vi "GUI.vi"() -> ()   [LabVIEW 2023]
uses:
  <vilib>/userDefined/High Color/IMAQdx.ctl
  <vilib>/vision/Image Controls.llb/IMAQ Image.ctl
  <vilib>/vision/Avi.llb/IMAQ AVI2 Refnum.ctl
  <vilib>/vision/driver/IMAQdx.llb/IMAQdx Acquisition Mode.ctl
  <vilib>/vision/driver/IMAQdx.llb/IMAQdx Buffer Number Mode.ctl
  <vilib>/Utility/error.llb/DialogType.ctl
  <vilib>/DAQmx/write.llb/DAQmx Write (Analog 1D Wfm NChan NSamp).vi
  <extravilib>/ChannelInstances/Tag-bool/Read With Abort.vi
  <extravilib>/ChannelInstances/Tag-t'IMAQ Image.ctl'/Read With Abort.vi
  <extravilib>/ChannelInstances/Messenger-str/Write With Abort.vi
  <extravilib>/ChannelInstances/Tag-str/Read With Abort.vi
  <extravilib>/ChannelInstances/Messenger-str/Read With Abort.vi
  <extravilib>/ChannelInstances/Tag-str/Write With Abort.vi
  <extravilib>/ChannelInstances/Tag-bool/Write With Abort.vi
  <extravilib>/ChannelInstances/Messenger-c(bool,i32,str)/Read With Abort.vi
  <extravilib>/ChannelInstances/Tag-c(bool,i32,str)/Write With Abort.vi
  <extravilib>/ChannelInstances/Tag-c(bool,i32,str)/Read With Abort.vi
  <extravilib>/ChannelInstances/Messenger-c(bool,i32,str)/Write With Abort.vi
  <vilib>/Utility/High Resolution Relative Seconds.vi
  <extravilib>/ChannelInstances/Tag-t'IMAQ Image.ctl'/Write With Abort.vi
  <extravilib>/ChannelInstances/Tag-str/Instantiate.vi
  <extravilib>/ChannelInstances/Messenger-str/Instantiate.vi
  <vilib>/DAQmx/create/channels.llb/DAQmx Create Channel (AO-Voltage-Basic).vi
  <vilib>/DAQmx/configure/timing.llb/DAQmx Timing (Sample Clock).vi
  <vilib>/DAQmx/configure/trigger.llb/DAQmx Start Trigger (Digital Edge).vi
  <vilib>/DAQmx/miscellaneous.llb/DAQmx Fill In Error Info.vi
  <extravilib>/ChannelInstances/Messenger-str/Endpoint.vi
  <extravilib>/ChannelInstances/Tag-str/EndpointRead.vi
  <extravilib>/ChannelInstances/Tag-str/Endpoint.vi
  <extravilib>/ChannelInstances/Tag-bool/Instantiate.vi
  <extravilib>/ChannelInstances/Tag-bool/Endpoint.vi
  <extravilib>/ChannelInstances/Tag-t'IMAQ Image.ctl'/Instantiate.vi
  <extravilib>/ChannelInstances/Tag-bool/EndpointRead.vi
  <extravilib>/ChannelInstances/Tag-t'IMAQ Image.ctl'/EndpointRead.vi
  <extravilib>/ChannelInstances/Tag-c(bool,i32,str)/Instantiate.vi
  <extravilib>/ChannelInstances/Messenger-c(bool,i32,str)/Instantiate.vi
  <extravilib>/ChannelInstances/Messenger-c(bool,i32,str)/Endpoint.vi
  <extravilib>/ChannelInstances/Tag-c(bool,i32,str)/Endpoint.vi
  <extravilib>/ChannelInstances/Tag-c(bool,i32,str)/EndpointRead.vi
  <vilib>/vision/EDVR.llb/IMAQ ImageToEDVR.vi
  <vilib>/vision/EDVR.llb/IMAQ ImageToEDVR 1D U8.vi
  <vilib>/vision/EDVR.llb/IMAQ ImageToEDVR 1D I16.vi
  <vilib>/vision/EDVR.llb/IMAQ ImageToEDVR 1D U32.vi
  <vilib>/vision/EDVR.llb/IMAQ ImageToEDVR 1D U16.vi
  <extravilib>/ChannelInstances/Tag-t'IMAQ Image.ctl'/Endpoint.vi
  <vilib>/vision/driver/NI_Vision_Acquisition_Software.lvlib
  <resource>/objmgr/imaqdx.rc
  <extravilib>/ChannelInstances/Messenger-str.lvlib
  <extravilib>/ChannelInstances/Messenger-c(bool,i32,str).lvlib
  <extravilib>/ChannelInstances/Tag-c(bool,i32,str).lvlib
  <extravilib>/ChannelInstances/Tag-t'IMAQ Image.ctl'.lvlib
  <extravilib>/ChannelInstances/Tag-bool.lvlib
  <resource>/objmgr/daqmx.rc
  <extravilib>/ChannelInstances/Tag-str.lvlib
  Control2.ctl
panel:
  in  "error IO":errorcluster
  in  "Stop 7":bool
  in  "Stop 6":bool
  in  "Stop 5":bool
  in  "Stop 4":bool
  in  "Stop 3":bool
  in  "Stop 2":bool
  in  "Stop":bool
  in  "Save Name":string
  in  "Save Path":path
  in  "Save Config":bool
  in  "Apply Configuration":bool
  in  "Config Path":path
  in  "Initialize from config file?":bool caption="Checkbox"
  in  "Quit":bool
  in  "Clock Button":bool
  in  "Controls":bool
  in  "Inputs":bool
  in  "Outputs":bool
  in  "Camera Setup":bool
  out "Tab Control":T1(tab)
  out "Sensor Readout Time":dbl
  out "Max FPS":dbl
  out "FPS":dbl
  out "Images Behind":dbl
  out "Missed Images":dbl
  out "Video Bytes/s":dbl
  out "Estimated Time":dbl
  in  "Initialize Camera":bool
  in  "Cluster - Borderless":T3={"Cluster - Borderless"={"Time Stamp\n Position"=enum."Exposure Center", "Frame rate Multiple of \nData Acquisition Rate"=FALSE}, "Sensor readout mode\n(Fast Decreases Quality)"=enum."Normal", "Pixel Format\n(p not supported)"=enum."Mono 10 p", "Gain"=0.0, "Gamma"=1.0, "Temporary Format\n(can be converted)"=enum."AVI", "Cluster - Borderless 2"={"Frame Limit"=0.0}, "Cluster - Borderless 3"={"Frame Limit"=0.0}, "Camera Ref"="", "Tempory Storage Location\n(File can be moved after acquisition)\nSSD recomended for high frame rate"=path "", "Images Per File"=0.0, "Buffer Images"=0.0, "Update Viewport Every N Frames"=0.0, "Exposure (ms)"=0.0, "FPS"=150.0, "Encoding Quality"=0.0, "Camera Signal Output Port"="", "Image Width"=0.0, "Image Height"=0.0, "Signal Line"=0, "Codec"=0, "Confirm File Write Optimizations (TDMS)"=FALSE, "Confirm Disable Buffering (advanced TDMS)"=FALSE} {"Codec" items=["(Select at runtime)", "YUV 4:2:0 Planar (NI Vision)", "Y800 Uncompressed Grey Scale (Ni Vision)", "VP9 (Ni Vision)", "Motion JPEG (NI Vision)", "FF Video Codec 1 (FFV1) (NI Vision)", "VP8 (NI Vision)"]; "Gamma" min=0.0 max=4.0 step=1.0 scale=0.0..3.0; "Gain" min=0.0 max=12.0092 step=1.0 scale=0.0..12.0}
  in  "Channel Names":string[](array[string])
  in  "XY Plot 2":cluster{"Ring - Menu":u16, "Ring - Menu 2":u16}
  in  "XY Plot 1":cluster{"Ring - Menu":u16, "Ring - Menu 2":u16}
  in  "Plot 4 Options":cluster{"Camera Signal":bool}
  in  "Plot 3 Options":cluster{"Camera Signal":bool}
  in  "Plot 2 Options":cluster{"Camera Signal":bool}
  in  "Plot 1 Options":cluster{"Camera Signal":bool}
  in  "Sample Buffer":dbl
  in  "Sample Rate":dbl
  in  "Input Channels":tag
  in  "Voltage Input Channel":tag
  in  "Current Input Channel":tag
  in  "Using Gamry Potentiostat":bool caption="Checkbox"
  in  "FPS 3":dbl=150.0
  out "FPS 2":dbl
  out "Images Behind 2":dbl
  out "Missed Images 2":dbl
  out "Estimated Time 2":dbl
  in  "Save Video":bool
  in  "Stop Acquisition":bool
  in  "Initialize Camera":bool
  in  "Outputs":T4
  in  "Re/Start Acquisition":bool
  in  "Exposure (ms)":dbl
  in  "Update Viewport Every N Frames":dbl
  in  "PlotSelector":T5(tab)
  in  "OneSelection":u16(ring) items=["None", "CameraDisplay", "Plot1", "Plot2", "Plot3", "Plot4", "XY1", "XY2"]
  in  "TwoVertSelL":u16(ring) items=["None", "CameraDisplay", "Plot1", "Plot2", "Plot3", "Plot4", "XY1", "XY2"]
  in  "TwoVertSelR":u16(ring) items=["None", "CameraDisplay", "Plot1", "Plot2", "Plot3", "Plot4", "XY1", "XY2"]
  in  "2HorizSelB":u16(ring) items=["None", "CameraDisplay", "Plot1", "Plot2", "Plot3", "Plot4", "XY1", "XY2"]
  in  "2HorizSelT":u16(ring) items=["None", "CameraDisplay", "Plot1", "Plot2", "Plot3", "Plot4", "XY1", "XY2"]
  in  "3PaneVertSelBR":u16(ring) items=["None", "CameraDisplay", "Plot1", "Plot2", "Plot3", "Plot4", "XY1", "XY2"]
  in  "3PaneVertSelTR":u16(ring) items=["None", "CameraDisplay", "Plot1", "Plot2", "Plot3", "Plot4", "XY1", "XY2"]
  in  "3PaneVertSelL":u16(ring) items=["None", "CameraDisplay", "Plot1", "Plot2", "Plot3", "Plot4", "XY1", "XY2"]
  in  "3PaneHorizBL":u16(ring) items=["None", "CameraDisplay", "Plot1", "Plot2", "Plot3", "Plot4", "XY1", "XY2"]
  in  "3PaneHorizBR":u16(ring) items=["None", "CameraDisplay", "Plot1", "Plot2", "Plot3", "Plot4", "XY1", "XY2"]
  in  "3PaneHorizT":u16(ring) items=["None", "CameraDisplay", "Plot1", "Plot2", "Plot3", "Plot4", "XY1", "XY2"]
  in  "4PaneSelBR":u16(ring) items=["None", "CameraDisplay", "Plot1", "Plot2", "Plot3", "Plot4", "XY1", "XY2"]
  in  "4PaneSelBL":u16(ring) items=["None", "CameraDisplay", "Plot1", "Plot2", "Plot3", "Plot4", "XY1", "XY2"]
  in  "4PaneSelTR":u16(ring) items=["None", "CameraDisplay", "Plot1", "Plot2", "Plot3", "Plot4", "XY1", "XY2"]
  in  "4PaneSelTL":u16(ring) items=["None", "CameraDisplay", "Plot1", "Plot2", "Plot3", "Plot4", "XY1", "XY2"]
  # "Basic Camera Controls"
  # "Camera"
  # "Image Aquisition Settings"
  # "Video File Settings"
  # "Advanced File Settings"
  # "Advanced Settings"
  # "(Must be multiple of 64)"
  # "AVI Settings"
  # "If very high framerates are required, save to TDMS not AVI\nFor high framerates Y800 is recomended, but requires\nconversion\nFor lower framerates, Motion JPEG saves \nspace and conversion time"
  # "For further advanced setting changes (binning,\netc.) open NI Max, select the camera, and change\nthe desired properties, pressing save at the end.\n\n(Note: This program may overwrite settings\ntemporarily while running in order to function)"
  # "(1-1000) or -1 for highest"
  # "Hardware Triggered\nAcquisition Settings"
  # "(Needs Reset)"
  # "Does not save video"
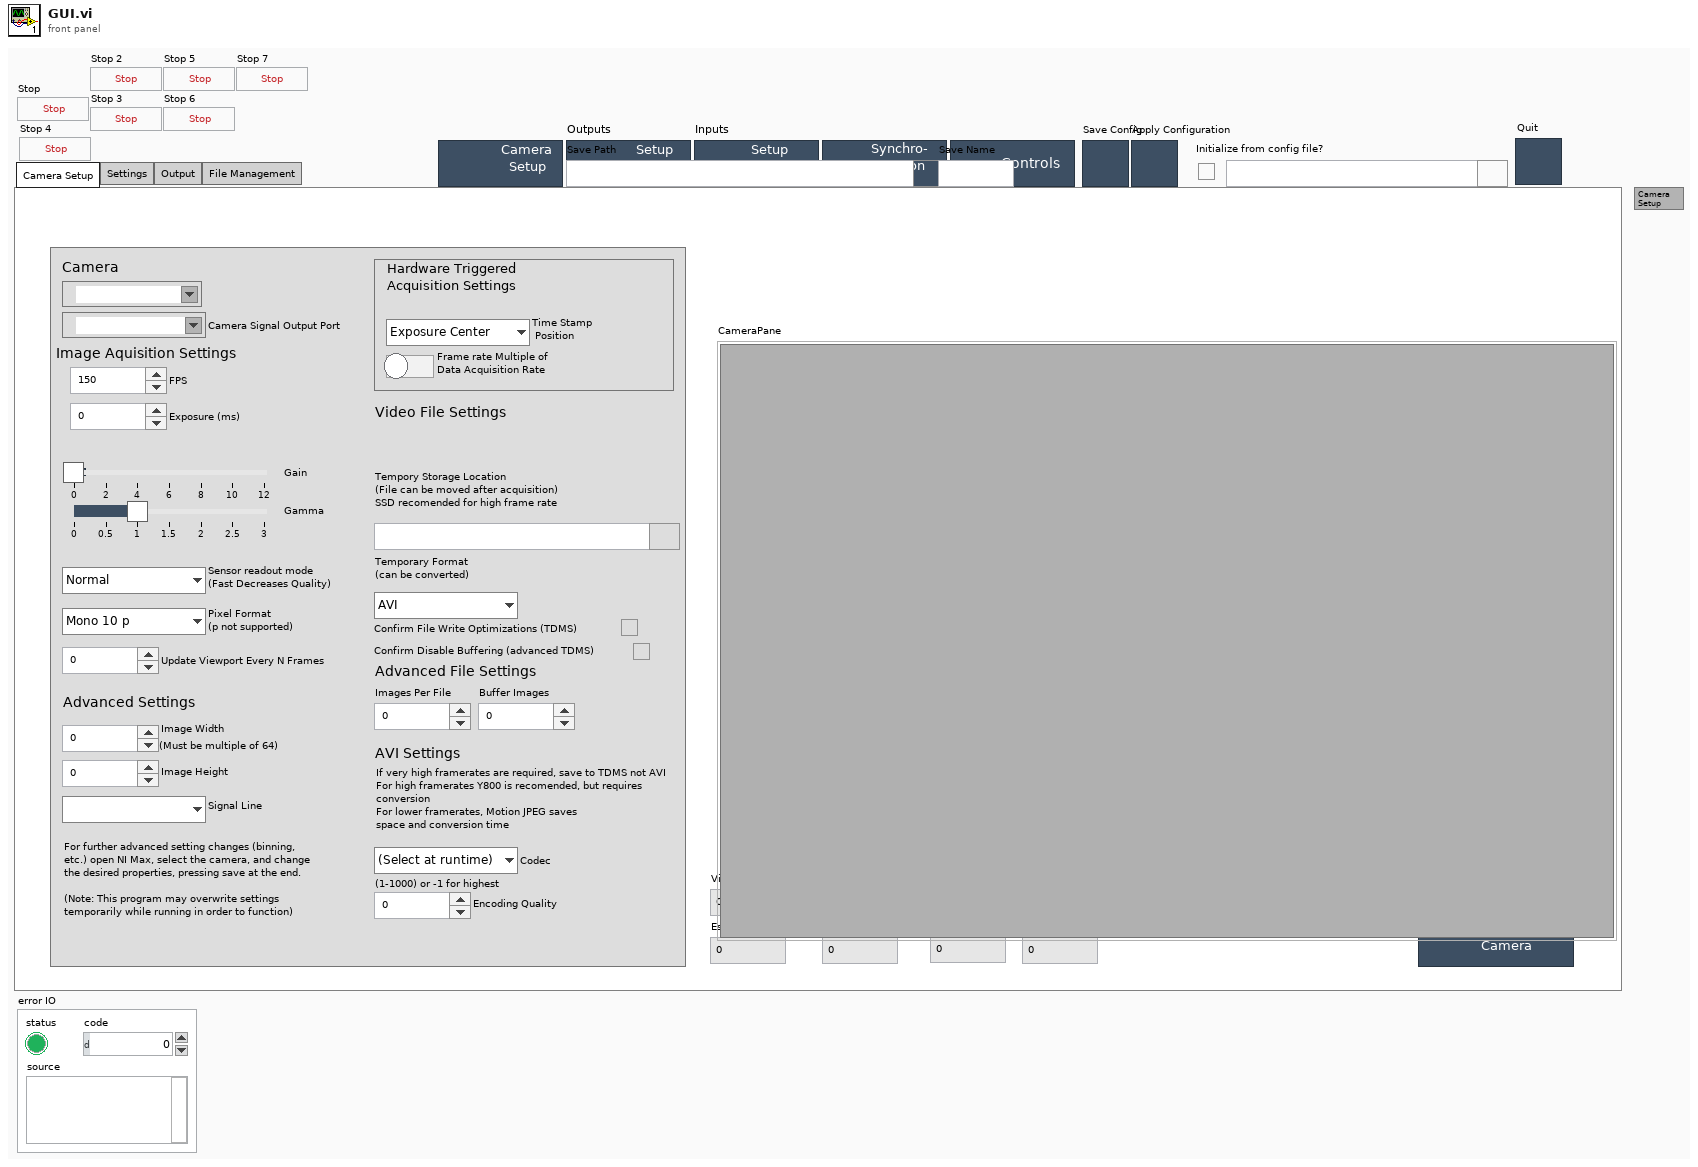
[diagram p1: front panel]
types:
  T1 = enum32{"Camera Setup", "Settings", "Output", "File Management"}
  T2 = typedef "IMAQdx.ctl" = refnum<k21>
  T3 = cluster{"Cluster - Borderless":cluster{"Time Stamp\n Position":enum16{"Exposure Center", "Exposure Beginning", "Exposure End"}, "Frame rate Multiple of \nData Acquisition Rate":bool}, "Sensor readout mode\n(Fast Decreases Quality)":enum16{"Normal", "Fast"}, "Pixel Format\n(p not supported)":enum16{"Mono 10 p", "Mono 10", "Mono 8"}, "Gain":dbl, "Gamma":dbl, "Temporary Format\n(can be converted)":enum16{"AVI", "TDMS", "None"}, "Cluster - Borderless 2":cluster{"Frame Limit":dbl}, "Cluster - Borderless 3":cluster{"Frame Limit":dbl}, "Camera Ref":T2, "Tempory Storage Location\n(File can be moved after acquisition)\nSSD recomended for high frame rate":path, "Images Per File":dbl, "Buffer Images":dbl, "Update Viewport Every N Frames":dbl, "Exposure (ms)":dbl, "FPS":dbl, "Encoding Quality":dbl, "Camera Signal Output Port":tag, "Image Width":dbl, "Image Height":dbl, "Signal Line":u16, "Codec":u16, "Confirm File Write Optimizations (TDMS)":bool, "Confirm Disable Buffering (advanced TDMS)":bool}
  T4 = cluster{"AO0":cluster{"signal type":enum16{"Sine Wave", "Triangle Wave", "Square Wave", "Sawtooth Wave"}, "Frequency":dbl, "Amplitude":dbl, "Offset":dbl, "Phase":dbl, "Duty Cycle":dbl}, "AO0Enable":bool, "AO1":cluster{"signal type":enum16{"Sine Wave", "Triangle Wave", "Square Wave", "Sawtooth Wave"}, "Frequency":dbl, "Amplitude":dbl, "Offset":dbl, "Phase":dbl, "Duty Cycle":dbl}, "AO1Enable":bool, "AO2":cluster{"signal type":enum16{"Sine Wave", "Triangle Wave", "Square Wave", "Sawtooth Wave"}, "Frequency":dbl, "Amplitude":dbl, "Offset":dbl, "Phase":dbl, "Duty Cycle":dbl}, "AO3Enable":bool, "AO0Name":string, "AO1Name":string, "AO2Name":string}
  T5 = enum32{"One Pane", "2 Vertical Panes", "2 Horizontal Panes", "3 Panes Vert", "3 Panes Horiz", "Four Panes"}
  T6 = typedef "Control2.ctl" = cluster{"SubPanel":refnum<vi>, "Selector":refnum<vi>}
  T7 = cluster{"Panel2":cluster{"SubPanel":refnum<vi>, "Selector":refnum<vi>}, "Panel3":cluster{"SubPanel":refnum<vi>, "Selector":refnum<vi>}, "Panel4":cluster{"SubPanel":refnum<vi>, "Selector":refnum<vi>}}
  T8 = cluster{"PreviousInfo":cluster{"FinalSamplePhase":dbl, "LastTf":timestamp, "LastSelectedPhase":dbl}[], "SyncStart":bool, "Leader":bool, "NoDependants":i32}
  T9 = cluster{"Physical Settings":cluster{"physical channels":tag, "source":tag, "Start Trigger":tag, "StartTriggered":bool}, "OutputTask":refnum<k21>, "GenerationSettings":cluster{"NumberOfSamples":i32, "Sample Rate":i32}, "Channel Names":string}
  T10 = cluster{"SyncStart":bool, "AfterErrorCheck":string, "SyncWait":bool, "VideoPath":path, "ConfirmTDMSOptimizations":bool, "ConfirmTDMSDisableBuffer":bool, "CameraOpen":bool, "TriggerStarted":bool, "AcquisitionStarted":bool, "FileOpen":bool, "VideoSave":bool, "BufferOpen":bool, "ShutdownActions":string[], "Acquisition Configured":bool}
  T11 = typedef "IMAQ Image.ctl" = refnum<image>
  T12 = typedef "IMAQ AVI2 Refnum.ctl" = refnum<k20>
  T13 = typedef "Image Type" = u32
  T14 = cluster{"User Camera Settings":cluster{"Pixel Format":string, "Width":i64, "Height":i64, "Trigger Source":string, "Readout Mode":string, "Session In":T2}, "IMAQdx Session":T2, "Trigger Settings":cluster{"FPS":i32, "Exposure Time":dbl, "Start Trigger Source":tag, "Camera\nClock\nCounter":tag, "PhysicalCameraSignalLine":tag, "Sync Type":enum16{"Exposure End", "Exposure Center", "Exposure Start", "Start", "NoSync"}}, "Camera Aq Attributes":cluster{"Readout Time":dbl, "Resulting FPS":dbl, "Width":u32, "Height":u32, "Format":u32, "Bit Depth":u32}, "Camera Attributes":cluster{"Exposure Start Delay":dbl}, "AcquisitionSettings":cluster{"Buffer":i32, "FramesPerFile":i32}, "Image Buffer":T11[], "Example Image":T11, "FileSettings":cluster{"FileSaveLocation":path, "FileName":string, "VideoSuffix":string, "Codec":string, "Quality":i32, "Format":string, "AVI FPS":i32}, "AVIRef":T12, "TDMSRef":refnum<k34>, "TDMSWSet":cluster{"Image Type":T13, "Async File Format":bool}, "CameraSignalRefnum":refnum<k21>, "CameraSignalDefinition":cluster{"High Time":dbl, "Low Time":dbl, "Delay":dbl}, "DisplayEveryNFrames":i32}
  T15 = typedef "Tag-bool.lvlib/))Channel.ctl" = refnum<queue>
  T16 = enum8{"Enabled", "Disabled", "Disabled and Grayed Out"}
  T17 = typedef "NI_Vision_Acquisition_Software.lvlib/IMAQdx Acquisition Mode.ctl" = enum32{"One Shot", "Continuous"}
  T18 = typedef "NI_Vision_Acquisition_Software.lvlib/IMAQdx Buffer Number Mode.ctl" = enum32{"Next", "Last", "Buffer Number", "Every", "Last New"}
  T19 = cluster{"Pixel Format":string, "Width":i64, "Height":i64, "Trigger Source":string, "Readout Mode":string, "Session In":T2}
  T20 = cluster{"Readout Time":dbl, "Resulting FPS":dbl, "Width":u32, "Height":u32, "Format":u32, "Bit Depth":u32}
  T21 = cluster{"FPS":i32, "Exposure Time":dbl, "Start Trigger Source":tag, "Camera\nClock\nCounter":tag, "PhysicalCameraSignalLine":tag, "Sync Type":enum16{"Exposure End", "Exposure Center", "Exposure Start", "Start", "NoSync"}}
  T22 = cluster{"FileSaveLocation":path, "FileName":string, "VideoSuffix":string, "Codec":string, "Quality":i32, "Format":string, "AVI FPS":i32}
  T23 = cluster{"Image Type":T13, "Async File Format":bool}
  T24 = cluster{"Asynchronous Writes":bool, "Reserve Disk Space":bool, "Disable Buffering":bool}
  T25 = typedef "Messenger-c(bool,i32,str).lvlib/))Channel.ctl" = refnum<queue>
  T26 = enum16{"Exposure End", "Exposure Center", "Exposure Start", "Start", "NoSync"}
  T27 = cluster{"High Time":dbl, "Low Time":dbl, "Delay":dbl}
  T28 = typedef "Messenger-str.lvlib/))Channel.ctl" = refnum<queue>
  T29 = typedef "DialogType.ctl" = u16
  T30 = typedef "Tag-t'IMAQ Image.ctl'.lvlib/))Channel.ctl" = refnum<queue>
  T31 = cluster{"physical channels":tag, "source":tag, "Start Trigger":tag, "StartTriggered":bool}
  T32 = cluster{"FinalSamplePhase":dbl, "LastTf":timestamp, "LastSelectedPhase":dbl}[]
  T33 = cluster{"AO0":cluster{"signal type":enum16{"Sine Wave", "Triangle Wave", "Square Wave", "Sawtooth Wave"}, "Frequency":dbl, "Amplitude":dbl, "Offset":dbl, "Phase":dbl, "Duty Cycle":dbl}, "AO0Enable":bool, "AO1":cluster{"signal type":enum16{"Sine Wave", "Triangle Wave", "Square Wave", "Sawtooth Wave"}, "Frequency":dbl, "Amplitude":dbl, "Offset":dbl, "Phase":dbl, "Duty Cycle":dbl}, "AO1Enable":bool, "AO2":cluster{"signal type":enum16{"Sine Wave", "Triangle Wave", "Square Wave", "Sawtooth Wave"}, "Frequency":dbl, "Amplitude":dbl, "Offset":dbl, "Phase":dbl, "Duty Cycle":dbl}, "AO3Enable":bool, "Nme":string, "Nme 2":string, "Nme 3":string}
  T34 = typedef "Tag-str.lvlib/))Channel.ctl" = refnum<queue>
  T35 = typedef "Tag-c(bool,i32,str).lvlib/))Channel.ctl" = refnum<queue>
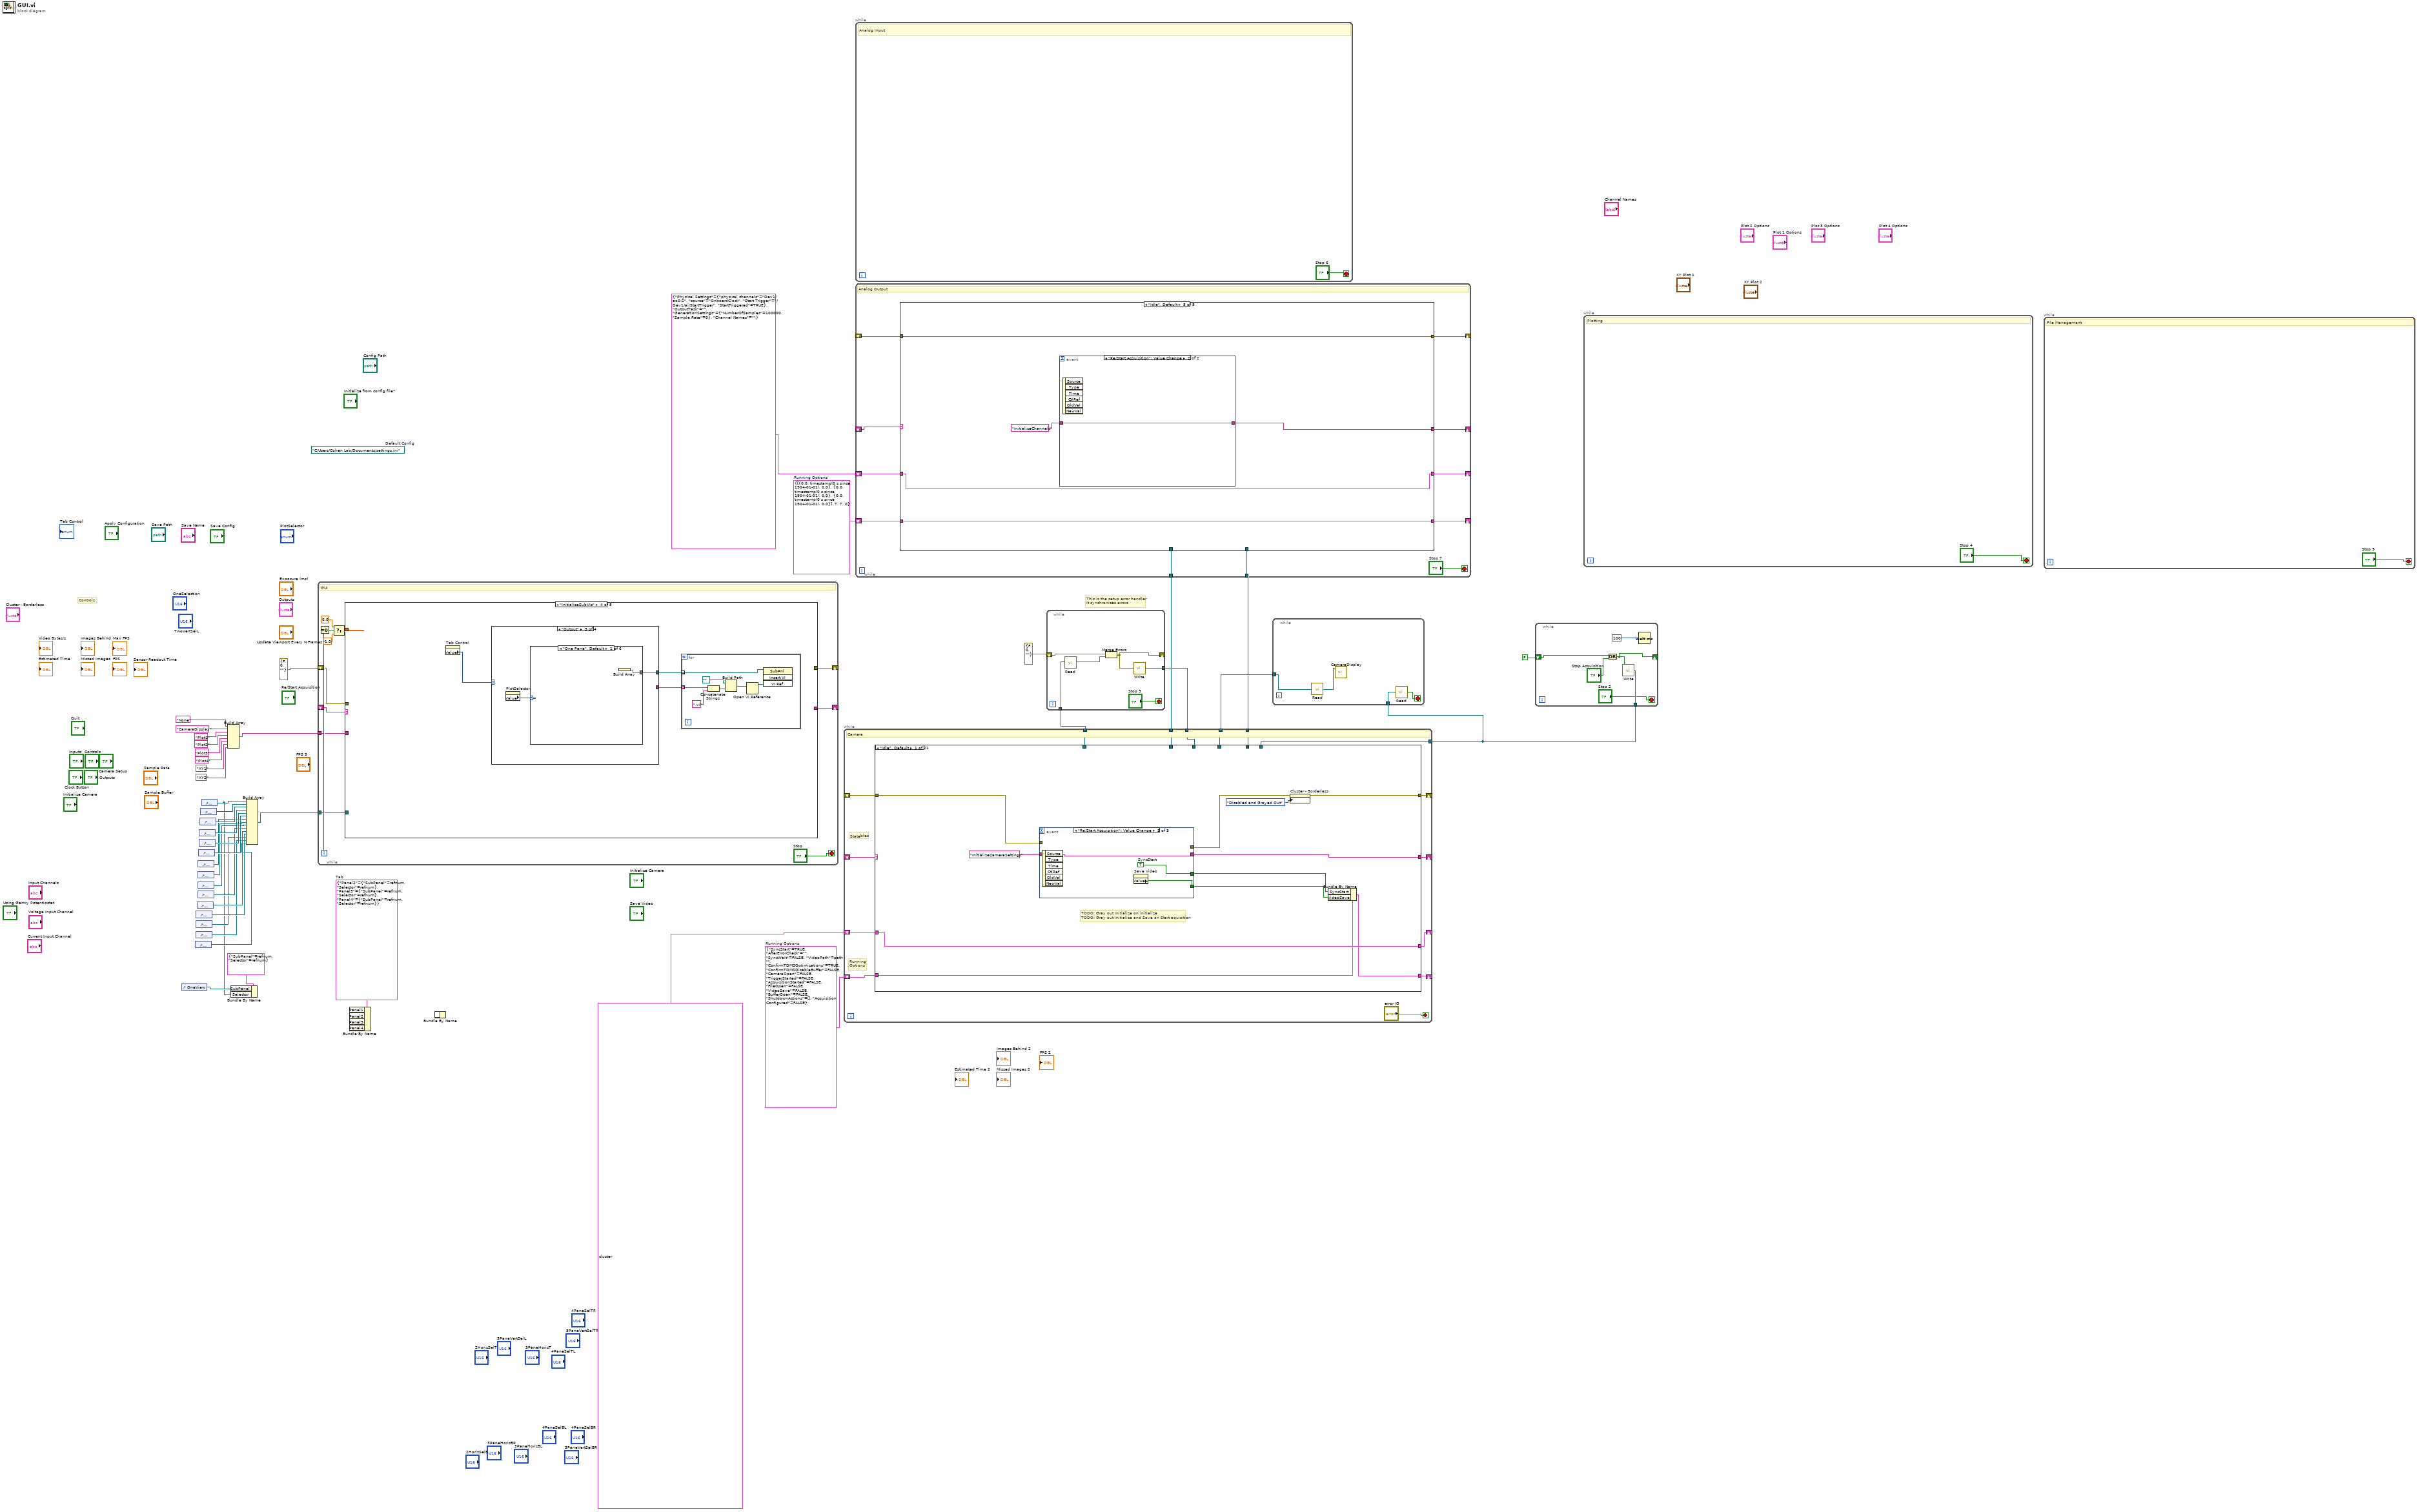
[diagram p0: block diagram]
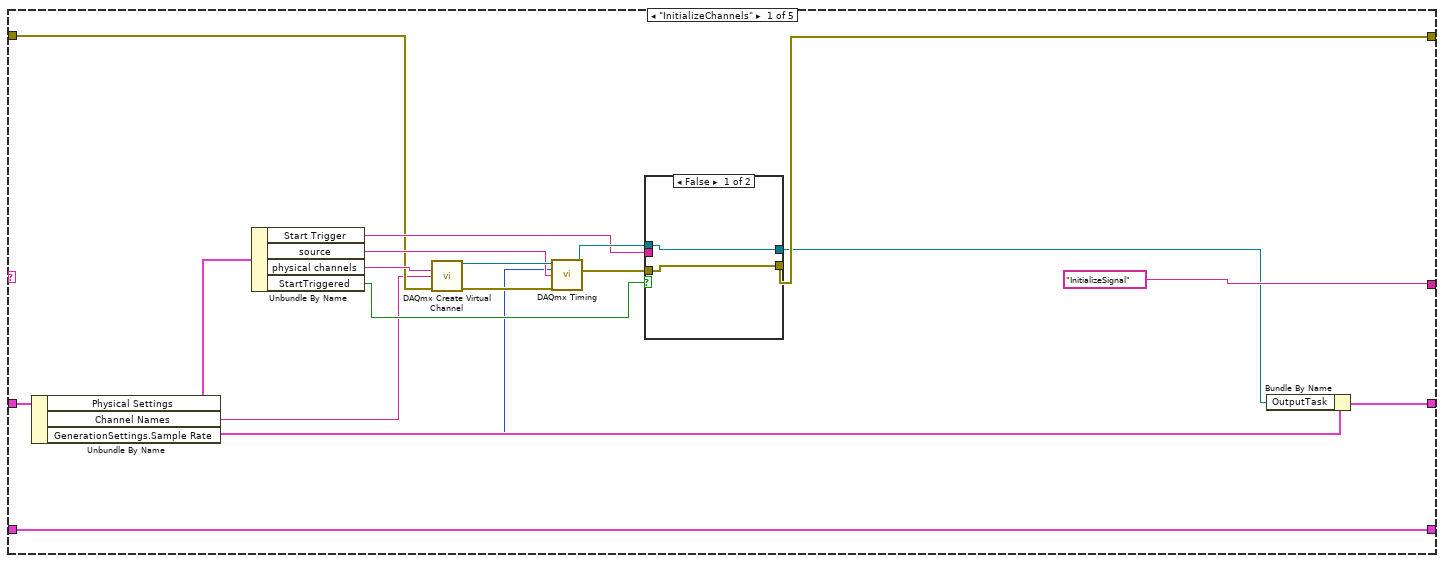
[diagram p2: hidden frame]
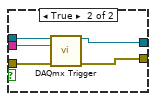
[diagram p3: hidden frame]
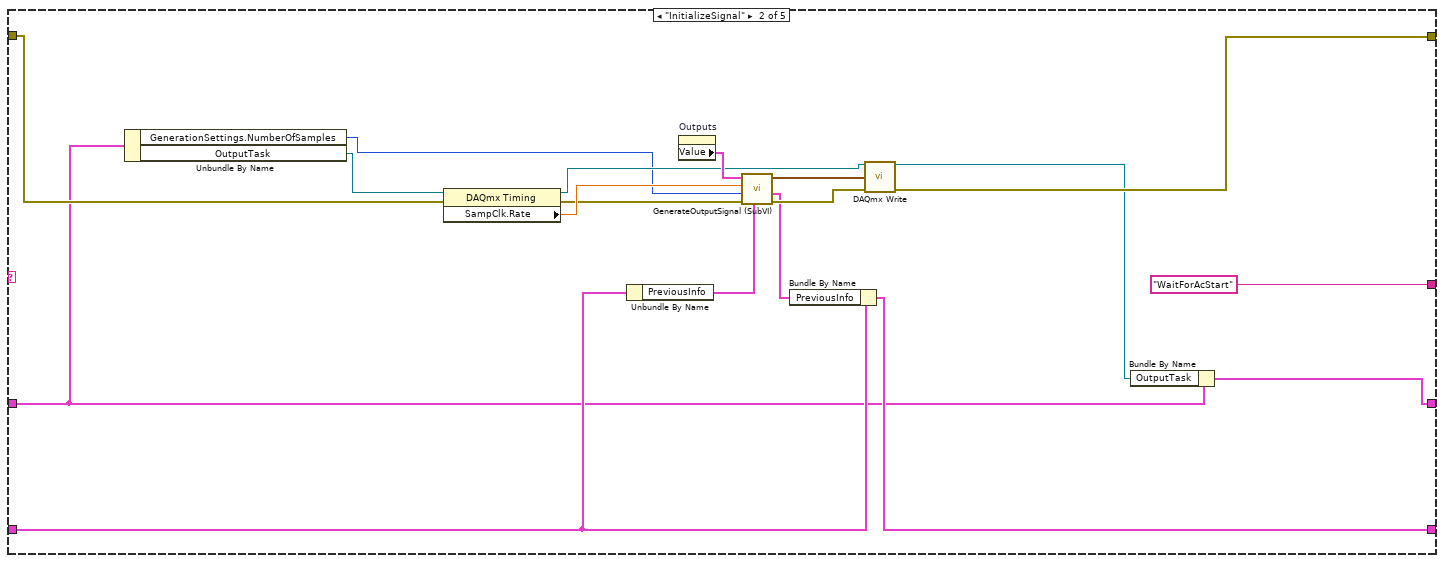
[diagram p4: hidden frame]
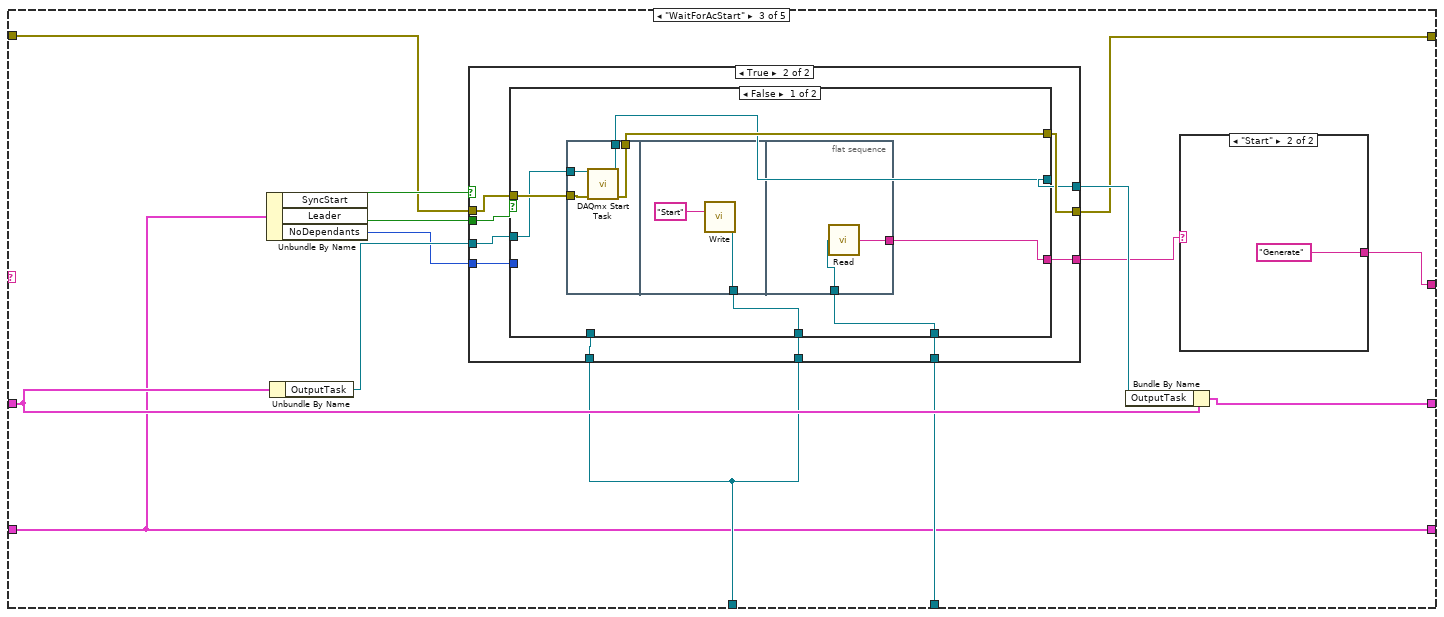
[diagram p5: hidden frame]
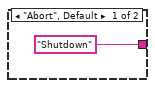
[diagram p6: hidden frame]
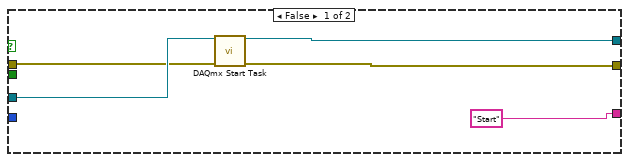
[diagram p7: hidden frame]
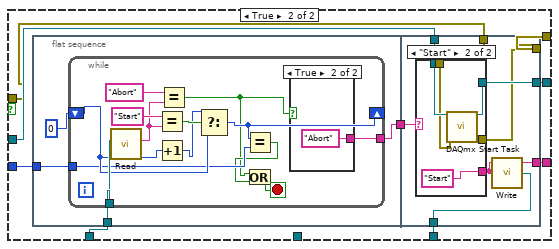
[diagram p8: hidden frame]
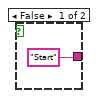
[diagram p9: hidden frame]
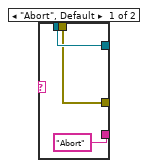
[diagram p10: hidden frame]
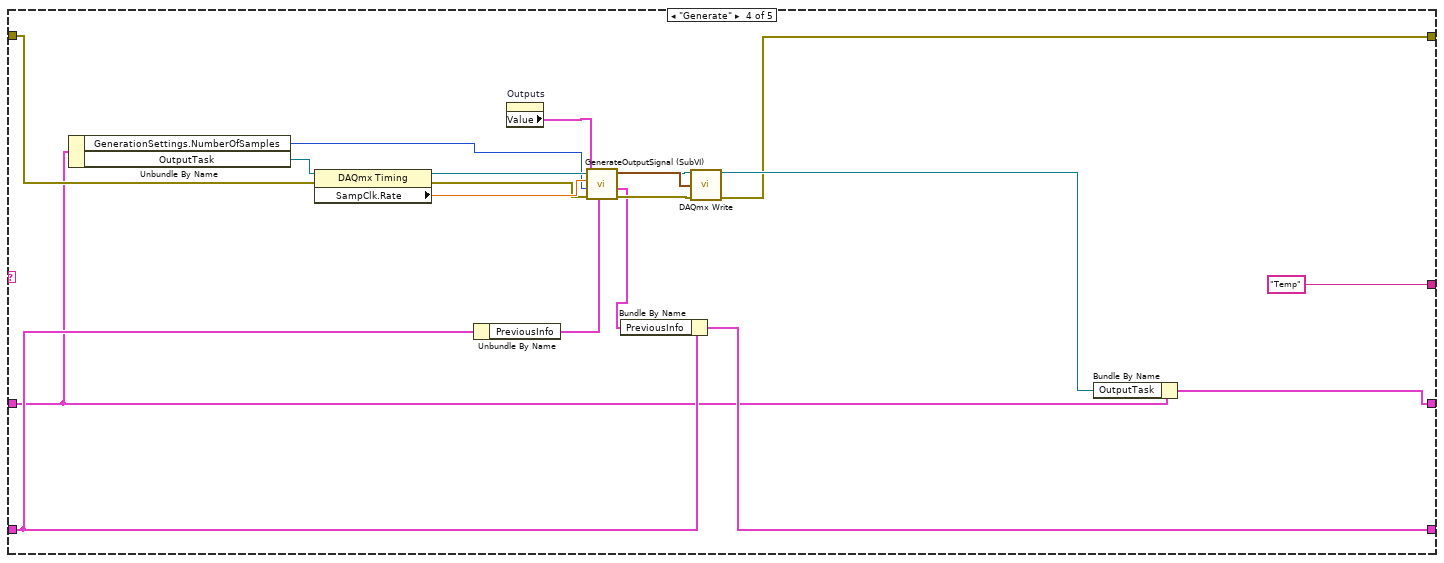
[diagram p11: hidden frame]
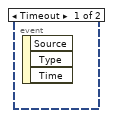
[diagram p12: hidden frame]
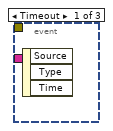
[diagram p13: hidden frame]
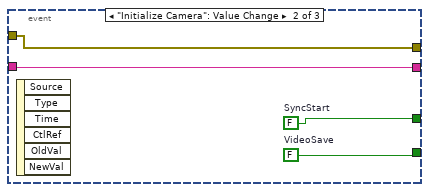
[diagram p14: hidden frame]
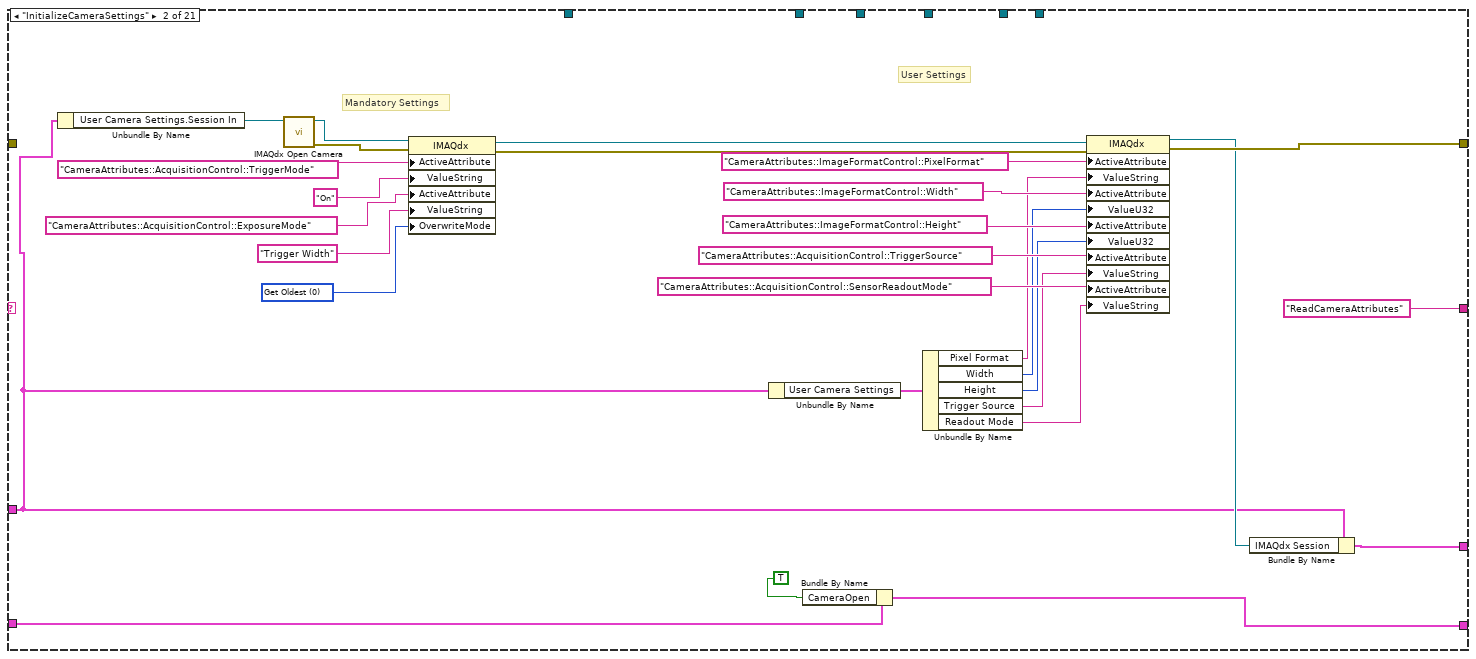
[diagram p15: hidden frame]
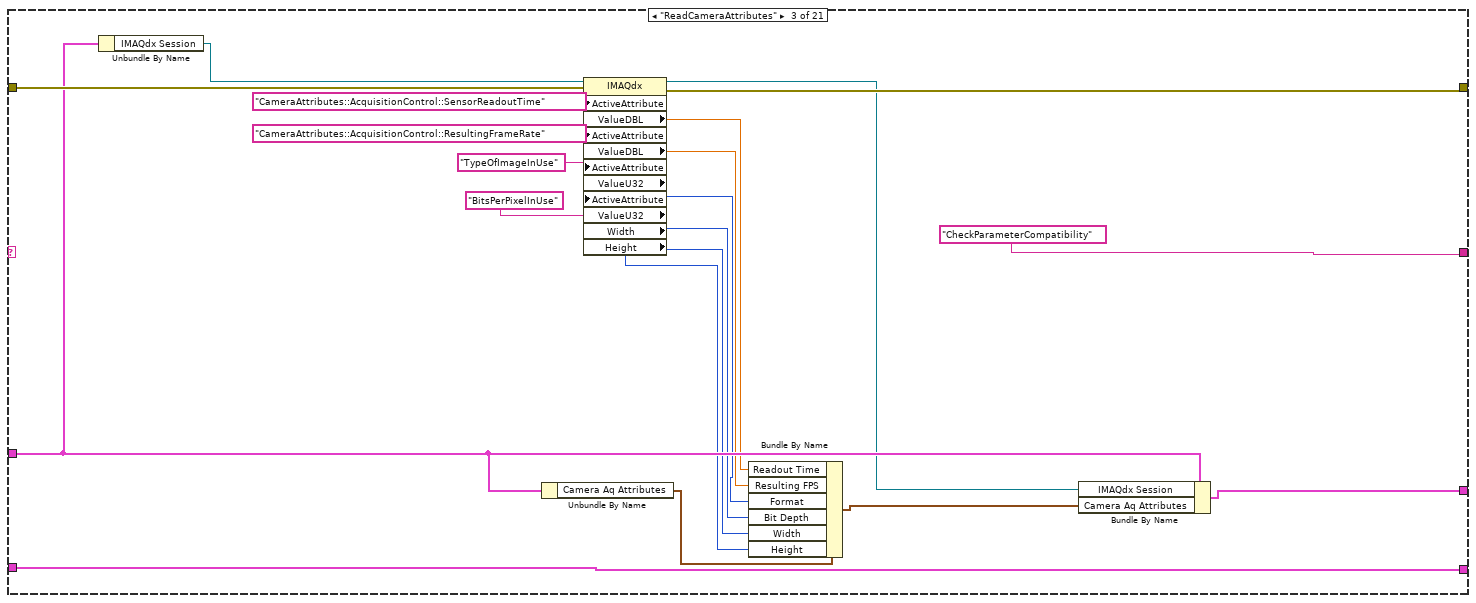
[diagram p16: hidden frame]
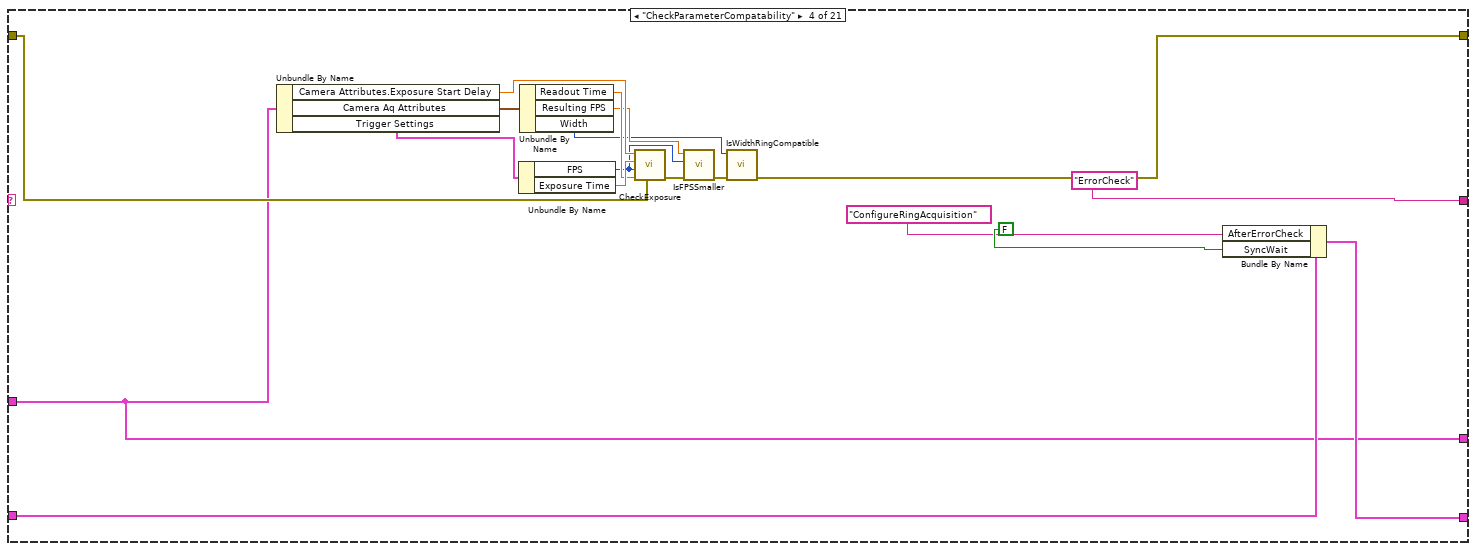
[diagram p17: hidden frame]
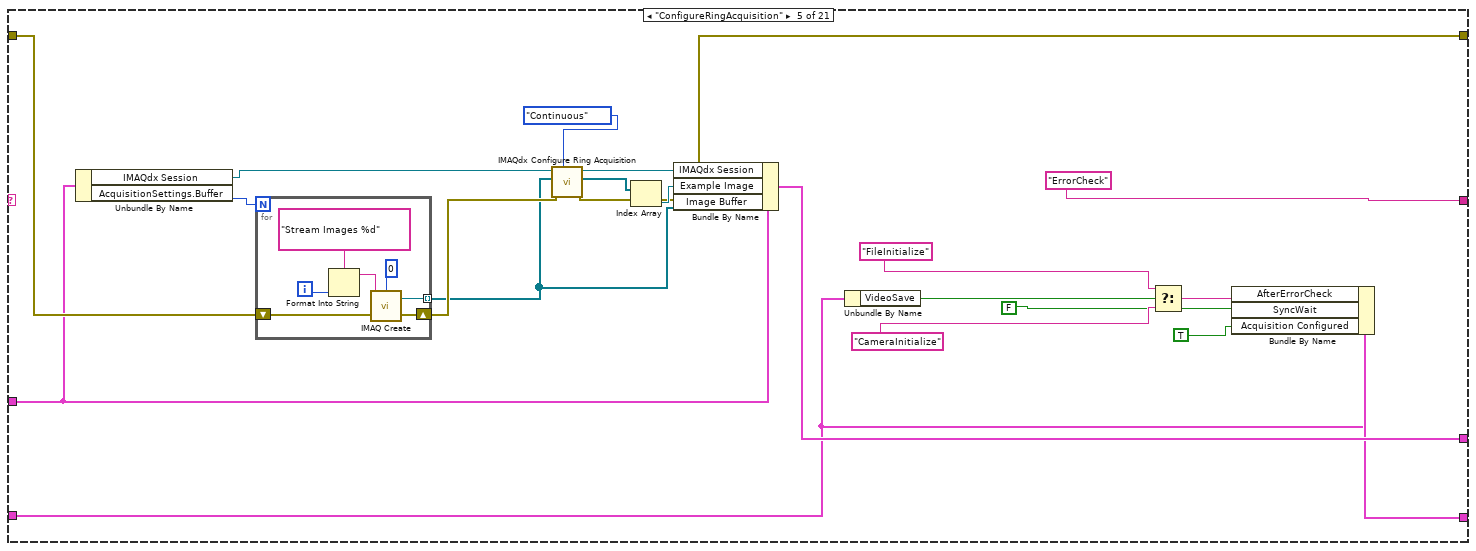
[diagram p18: hidden frame]
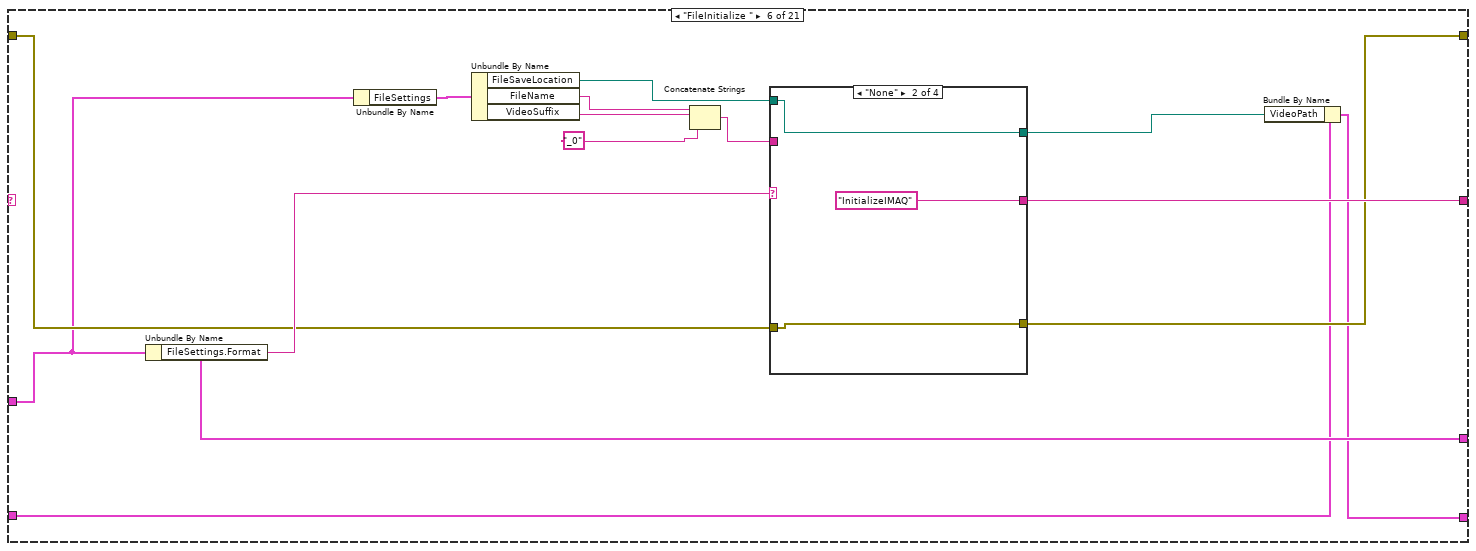
[diagram p19: hidden frame]
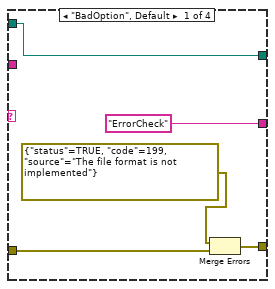
[diagram p20: hidden frame]
diagram:
  w4 = T7 {"Panel2"={"SubPanel"=refnum, "Selector"=refnum}, "Panel3"={"SubPanel"=refnum, "Selector"=refnum}, "Panel4"={"SubPanel"=refnum, "Selector"=refnum}}  # Tab
  w32 = T8 {"PreviousInfo"=[{"FinalSamplePhase"=0.0, "LastTf"=timestamp(0 s since 1904-01-01), "LastSelectedPhase"=0.0}, {"FinalSamplePhase"=0.0, "LastTf"=timestamp(0 s since 1904-01-01), "LastSelectedPhase"=0.0}, {"FinalSamplePhase"=0.0, "LastTf"=timestamp(0 s since 1904-01-01), "LastSelectedPhase"=0.0}], "SyncStart"=TRUE, "Leader"=TRUE, "NoDependants"=0}  # Running Options
  w40 = T10 {"SyncStart"=TRUE, "AfterErrorCheck"="", "SyncWait"=FALSE, "VideoPath"=path "", "ConfirmTDMSOptimizations"=TRUE, "ConfirmTDMSDisableBuffer"=FALSE, "CameraOpen"=FALSE, "TriggerStarted"=FALSE, "AcquisitionStarted"=FALSE, "FileOpen"=FALSE, "VideoSave"=FALSE, "BufferOpen"=FALSE, "ShutdownActions"=[], "Acquisition Configured"=FALSE}  # Running Options
  (unwired) path "C:/Users/Cohen Lab/Documents/settings.ini"  # Default Config
  # "This is the setup error handler\nIt synchronizes errors"
  # "Controls"
  n1 = control-ref of="OneView"() -> (w2:refnum<vi>)
  n2 = control-ref of="4PaneSelBR"() -> (w15:refnum<vi>)
  n3 = control-ref of="4PaneSelBL"() -> (w16:refnum<vi>)
  n4 = control-ref of="4PaneSelTL"() -> (w18:refnum<vi>)
  n5 = control-ref of="4PaneSelTR"() -> (w17:refnum<vi>)
  n6 = control-ref of="3PaneHorizBR"() -> (w19:refnum<vi>)
  n7 = control-ref of="3PaneVertSelBR"() -> (w22:refnum<vi>)
  n8 = control-ref of="3PaneHorizT"() -> (w21:refnum<vi>)
  n9 = control-ref of="3PaneHorizBL"() -> (w20:refnum<vi>)
  n10 = control-ref of="3PaneVertSelTR"() -> (w23:refnum<vi>)
  n11 = control-ref of="3PaneVertSelL"() -> (w24:refnum<vi>)
  n12 = control-ref of="2HorizSelT"() -> (w26:refnum<vi>)
  n13 = control-ref of="2HorizSelB"() -> (w25:refnum<vi>)
  n14 = control-ref of="TwoVertSelR"() -> (w27:refnum<vi>)
  n15 = control-ref of="TwoVertSelL"() -> (w28:refnum<vi>)
  n16 = control-ref of="OneSelection"() -> (w1:refnum<vi>)
  n17 = Build Array("None", "CameraDisplay", "Plot1", "Plot2", "Plot3", "Plot4", "XY1", "XY2") -> (w5:string[])
  n18 = Bundle By Name(cluster=T6 {"SubPanel"=refnum, "Selector"=refnum} ("Panel1"), "SubPanel"=w2, "Selector"=w1) -> ()  [unwired: 1 out]
  n19 = Build Array(w1, w28, w27, w26, w25, w24, w23, w22, w21, w20, w19, w18, w17, w16, w15) -> (w14:refnum<vi>[])
  n20 = while {
    shift-right: [w53] -> _
    shift-left: _ -> [w52]
    shift-right: [w46] -> _
    shift-left: errorcluster {"status"=FALSE, "code"=0, "source"=""} ("error constant") -> [w45]
    tunnel: w14 -> [w43]
    tunnel: w5 -> [w42]
    i -> [w51]
    stop <- "Stop" stop-if-true
    # "GUI"
    n21 = Equal To 0?(x=w51) -> (x = 0?=w50:bool)
    n22 = Select(t=0.0, s=w50, f=-1.0) -> (s? t:f=w47:dbl)
    n23 = case shown="\"InitializeSubVIs\"" w52 {
      tunnel: [w55 "InitializeSubViSelections" "InitializeSubVIs" _ "Temp"] -> w53
      tunnel: w47 -> [w56 _ _ _ _]
      tunnel: w45 -> [w54 w59 w63 _ w85]
      tunnel: [w54 w59 w63 _ w85] -> w46
      tunnel: w43 -> [_ _ w62 _ _]
      tunnel: w42 -> [_ _ w61 _ _]
      frame "Idle", Default {
        n24 = event shown="[1] \"PlotSelector\": Value Change" {
          selector: _ -> [_ _]
          dyn-events: _ -> [_ _]
          timeout: w56 -> [_ _]
          tunnel: ["Initialize" "UpdatePlotTab"] -> w55
          event Timeout {
            n25 = event-data() -> ()  [unwired: 1 in, 3 out]
          }
          event "PlotSelector": Value Change {
            n26 = event-data() -> ()  [unwired: 1 in, 6 out]
          }
        }
      }
      frame "Initialize" {
      }
      frame "InitializeSubViSelections" {
        n27 = for {
          tunnel: w62 -> [w66] mode=indexing
          tunnel: w61 -> [w65]
          n28 = property class="Ring (strict)"(reference=w66, "Strings []"=w65) -> ()  [unwired: 1 in, 2 out]
        }
      }
      frame "InitializeSubVIs" {
        n29 = property on="Tab Control" class="TabCtl (strict)"() -> ("Value"=w69:T1)  [unwired: 2 in, 2 out]
        n30 = case shown="\"Output\"" w69 {
          tunnel: [w79 _ _ _] -> w68
          tunnel: [w77 _ w81 _] -> w67
          frame "Camera Setup", Default {
            n31 = control-ref of="CameraPane"() -> (w78:refnum<vi>)
            n32 = Build Array(w78) -> (w77:refnum<vi>[])
            n33 = Build Array("CameraDisplay") -> (w79:string[])
          }
          frame "Settings" {
          }
          frame "Output" {
            n34 = property on="PlotSelector" class="TabCtl (strict)"() -> ("Value"=w82:T5)  [unwired: 2 in, 2 out]
            n35 = case shown="\"One Pane\", Default" w82 {
              tunnel: [w83 _ _ _ _ _] -> w81
              frame "One Pane", Default {
                n36 = Build Array() -> (w83:void[])  [unwired: 1 in]
              }
              frame "2 Vertical Panes" {
              }
              frame "2 Horizontal Panes" {
              }
              frame "3 Panes Vert" {
              }
              frame "3 Panes Horiz" {
              }
              frame "Four Panes" {
              }
            }
          }
          frame "File Management" {
          }
        }
        n37 = for {
          tunnel: w68 -> [w72] mode=indexing
          tunnel: w67 -> [w71] mode=indexing
          n38 = Concatenate Strings(w72, ".vi") -> (w75:string)
          n39 = Build Path(base path=path "", name or relative path=w75) -> (appended path=w73:path)
          n40 = Open VI Reference(vi path=w73) -> (vi reference=w70:refnum<vi>)  [unwired: 5 in, 1 out]
          n41 = invoke class="SubPnl" method="Insert VI"(reference=w71, "VI Ref"=w70) -> ()  [unwired: 2 in, 4 out]
        }
      }
      frame "UpdatePlotTab" {
        n42 = property on="PlotSelector" class="TabCtl (strict)" props=["Value"]() -> ()  [unwired: 2 in, 3 out]
      }
    }
  }
  n43 = Bundle By Name(cluster=w4) -> ()  [unwired: 4 in, 1 out]
  n44 = Bundle By Name() -> ()  [unwired: 2 in, 1 out]
  n45 = while {
    stop <- "Stop 6" stop-if-true
    # "Analog Input"
  }
  n46 = while {
    shift-right: [w92] -> _
    shift-left: FALSE -> [w90]
    tunnel: [w88] -> w35
    stop <- "Stop 2" stop-if-true
    n47 = Or(x=w90, y="Stop Acquisition") -> (x .or. y?=w92:bool)
    n48 = call <extravilib>:"Write.vi"("element"=w92) -> ("channel"=w88:T15)  [unwired: 1 out]
    n49 = Wait (ms)(milliseconds to wait=u32 100) -> ()  [unwired: 1 out]
  }
  n50 = while {
    stop <- "Stop 4" stop-if-true
    # "Plotting"
  }
  n51 = while {
    stop <- "Stop 5" stop-if-true
    # "File Management"
  }
  n52 = while {
    shift-right: [w108] -> _
    shift-left: _ -> [w109]
    shift-right: [w106] -> _
    shift-left: T14 {"User Camera Settings"={"Pixel Format"="Mono 8", "Width"=704, "Height"=704, "Trigger Source"="Line 3", "Readout Mode"="Normal", "Session In"="cam0"}, "IMAQdx Session"="", "Trigger Settings"={"FPS"=0, "Exposure Time"=0.0, "Start Trigger Source"="", "Camera\nClock\nCounter"="Dev1/ctr0", "PhysicalCameraSignalLine"="/Dev1/PFI2", "Sync Type"=enum."Exposure Center"}, "Camera Aq Attributes"={"Readout Time"=0.0, "Resulting FPS"=0.0, "Width"=0, "Height"=0, "Format"=0, "Bit Depth"=0}, "Camera Attributes"={"Exposure Start Delay"=0.0}, "AcquisitionSettings"={"Buffer"=0, "FramesPerFile"=0}, "Image Buffer"=[], "Example Image"=refnum, "FileSettings"={"FileSaveLocation"=path "", "FileName"="", "VideoSuffix"="", "Codec"="", "Quality"=0, "Format"="", "AVI FPS"=0}, "AVIRef"=refnum, "TDMSRef"=refnum, "TDMSWSet"={"Image Type"=0, "Async File Format"=FALSE}, "CameraSignalRefnum"="", "CameraSignalDefinition"={"High Time"=0.0, "Low Time"=0.0, "Delay"=0.0}, "DisplayEveryNFrames"=0} -> [w107]
    shift-right: [w105] -> _
    shift-left: _ -> [w104]
    shift-right: [w102] -> _
    shift-left: w40 -> [w103]
    tunnel: [w101] -> w39
    tunnel: w37 -> [w100]
    tunnel: [w99] -> w36
    tunnel: w35 -> [w98]
    tunnel: [w97] -> w31
    tunnel: w30 -> [w96]
    stop <- "error IO" stop-if-true
    # "State"
    # "Variables"
    # "Running\nOptions"
    # "Camera"
    n53 = case shown="\"Idle\", Default" w109 {
      tunnel: [w119 "ReadCameraAttributes" "CheckParameterCompatibility" "ErrorCheck" "ErrorCheck" ("AfterErrorCheck") w235 "ErrorCheck" ("AfterErrorCheck") "ErrorCheck" ("AfterErrorCheck") w334 "ErrorCheck" ("AfterErrorCheck") "WaitForAcStart" w378 w435 w548 "Shutdown" ("AfterErrorCheck") "Shutdown" ("AfterErrorCheck") "Shutdown" ("AfterErrorCheck") "Shutdown" ("AfterErrorCheck") "Shutdown" ("AfterErrorCheck") "Shutdown" ("AfterErrorCheck") "Idle" ("AfterErrorCheck")] -> w108
      tunnel: w107 -> [w118 w132 w170 w178 w210 w228 w270 w296 w337 w346 w360 w379 w413 w551 w583 w597 w606 w612 w633 w639 w650]
      tunnel: [w118 w135 w171 w178 w205 w228 w271 w293 w337 w347 w361 w383 w444 w551 w583 w596 w605 w612 w633 w639 w650] -> w106
      tunnel: [w111 w136 w160 w182 w206 w233 w268 w292 w332 w350 w362 w377 w415 w550 w584 w594 w603 w615 w631 w638 w646] -> w105
      tunnel: w104 -> [w113 _ w173 w192 w211 w234 w263 w313 w331 w351 w366 w385 w450 w550 w585 w595 w602 w616 w632 w638 w651]
      tunnel: w103 -> [w117 w129 w157 w180 w201 w225 w262 w308 w327 w352 w357 w382 w422 w546 w582 w592 w601 w611 w629 w637 w649]
      tunnel: [w115 w130 w157 w181 w202 w223 w266 w314 w326 w353 w357 w381 w421 w552 w581 w590 w601 w610 w627 w635 w649] -> w102
      tunnel: [_ _ _ _ _ _ _ _ w333 _ _ _ _ _ _ _ _ _ _ _ _] -> w101
      tunnel: w100 -> [_ _ _ _ _ _ _ _ w330 _ _ _ _ _ _ _ _ _ _ _ _]
      tunnel: [_ _ _ _ _ _ _ _ _ _ _ _ w437 _ _ _ _ _ _ _ _] -> w99
      tunnel: w98 -> [_ _ _ _ _ _ _ _ _ _ _ _ w433 _ _ _ _ _ _ _ _]
      tunnel: [_ _ _ _ _ _ _ _ _ _ _ w374 _ _ _ _ _ _ _ _ _] -> w97
      tunnel: w96 -> [_ _ _ _ _ _ _ _ _ _ _ w373 _ _ _ _ _ _ _ _ _]
      frame "Idle", Default {
        # "TODO: Gray out Initialize on initialize \nTODO: Gray out Initialize and Save on Start aquisition"
        n54 = event shown="[2] \"Re/Start Acquisition\": Value Change" {
          selector: _ -> [_ _ _]
          dyn-events: _ -> [_ _ _]
          timeout: _ -> [_ _ _]
          tunnel: [_ w124 w127] -> w119
          tunnel: "InitializeCameraSettings" -> [_ w124 w127]
          tunnel: [_ w123 w126] -> w116
          tunnel: [_ w122 w125] -> w114
          tunnel: w113 -> [_ w121 _]
          tunnel: [_ w121 _] -> w112
          event Timeout {
            n55 = event-data() -> ()  [unwired: 1 in, 3 out]
          }
          event "Initialize Camera": Value Change {
            w122 = FALSE  # VideoSave
            w123 = FALSE  # SyncStart
            n56 = event-data() -> ()  [unwired: 1 in, 6 out]
          }
          event "Re/Start Acquisition": Value Change {
            w126 = TRUE  # SyncStart
            n57 = event-data() -> ()  [unwired: 1 in, 6 out]
            n58 = property on="Save Video" class="Bool (strict)"() -> ("Value"=w125:bool)  [unwired: 2 in, 2 out]
          }
        }
        n59 = property on="Cluster - Borderless" class="Clust (strict)"(error in=w112, "DisabledEnum"=T16."Disabled and Grayed Out" ("Disabled")) -> (error out=w111:errorcluster)  [unwired: 1 in, 1 out]
        n60 = Bundle By Name(cluster=w117, "SyncStart"=w116, "VideoSave"=w114) -> (w115:T10)
      }
      frame "InitializeCameraSettings" {
        w133 = u32 0 items=["Get Oldest"=0, "Fail"=2, "Get Newest"=3] ("OverwriteMode")
        # "User Settings"
        # "Mandatory Settings"
        n61 = Unbundle By Name(w132) -> ("User Camera Settings.Session In"=w131:T2)
        n62 = call <vilib>:"IMAQdx Open Camera.vi"("Session In"=w131) -> ("error out"=w156:errorcluster, "Session Out"=w155:T2)  [unwired: 9 in]
        n63 = property class="IMAQdx"(reference=w155, error in=w156, "ActiveAttribute"="CameraAttributes::AcquisitionControl::TriggerMode", "ValueString"="On", "ActiveAttribute"="CameraAttributes::AcquisitionControl::ExposureMode", "ValueString"="Trigger Width", "OverwriteMode"=w133) -> (reference out=w150:T2, error out=w149:errorcluster)
        n64 = Unbundle By Name(w132) -> ("User Camera Settings"=w148:T19)
        n65 = Bundle By Name(cluster=w129, "CameraOpen"=TRUE) -> (w130:T10)
        n66 = Unbundle By Name(w148) -> ("Pixel Format"=w142:string, "Width"=w141:i64, "Height"=w140:i64, "Trigger Source"=w139:string, "Readout Mode"=w138:string)
        n67 = property class="IMAQdx"(reference=w150, error in=w149, "ActiveAttribute"="CameraAttributes::ImageFormatControl::PixelFormat", "ValueString"=w142, "ActiveAttribute"="CameraAttributes::ImageFormatControl::Width", "ValueU32"=w141, "ActiveAttribute"="CameraAttributes::ImageFormatControl::Height", "ValueU32"=w140, "ActiveAttribute"="CameraAttributes::AcquisitionControl::TriggerSource", "ValueString"=w139, "ActiveAttribute"="CameraAttributes::AcquisitionControl::SensorReadoutMode", "ValueString"=w138) -> (reference out=w134:T2, error out=w136:errorcluster)
        n68 = Bundle By Name(cluster=w132, "IMAQdx Session"=w134) -> (w135:T14)
      }
      frame "ReadCameraAttributes" {
        n69 = Unbundle By Name(w170) -> ("IMAQdx Session"=w174:T2)
        n70 = Unbundle By Name(w170) -> ("Camera Aq Attributes"=w169:T20)
        n71 = property class="IMAQdx"(reference=w174, error in=w173, "ActiveAttribute"="CameraAttributes::AcquisitionControl::SensorReadoutTime", "ActiveAttribute"="CameraAttributes::AcquisitionControl::ResultingFrameRate", "ActiveAttribute"="TypeOfImageInUse", "ActiveAttribute"="BitsPerPixelInUse") -> (reference out=w158:T2, error out=w160:errorcluster, "ValueDBL"=w168:dbl, "ValueDBL"=w167:dbl, "ValueU32"=w164:u32, "ValueU32"=w163:u32, "Width"=w162:u32, "Height"=w161:u32)
        n72 = Bundle By Name(cluster=w169, "Readout Time"=w168, "Resulting FPS"=w167, "Format"=w164, "Bit Depth"=w163, "Width"=w162, "Height"=w161) -> (w159:T20)
        n73 = Bundle By Name(cluster=w170, "IMAQdx Session"=w158, "Camera Aq Attributes"=w159) -> (w171:T14)
      }
      frame "CheckParameterCompatability" {
        n74 = Unbundle By Name(w178) -> ("Camera Attributes.Exposure Start Delay"=w191:dbl, "Camera Aq Attributes"=w188:T20, "Trigger Settings"=w190:T21)
        n75 = Unbundle By Name(w190) -> ("FPS"=w186:i32, "Exposure Time"=w189:dbl)
        n76 = Unbundle By Name(w188) -> ("Readout Time"=w187:dbl, "Resulting FPS"=w185:dbl, "Width"=w184:u32)
        n77 = call "CheckExposure.vi"("error constant"=w192, "Sensor readout time"=w187, "Frame Rate"=w186, "Exposure Time"=w189, "Exposure Start Delay"=w191) -> ("error out"=w194:errorcluster)  [unwired: 6 in]
        n78 = call "IsFPSSmaller.vi"("error constant"=w194, "Frame Rate"=w186, "Max FrameRate"=w185) -> ("error out"=w193:errorcluster)  [unwired: 8 in]
        n79 = call "IsWidthRingCompatible.vi"("error in (no error)"=w193, "Width"=w184) -> ("error out"=w182:errorcluster)  [unwired: 9 in]
        n80 = Bundle By Name(cluster=w180, "AfterErrorCheck"="ConfigureRingAcquisition", "SyncWait"=FALSE) -> (w181:T10)
      }
      frame "ConfigureRingAcquisition" {
        n81 = Unbundle By Name(w210) -> ("IMAQdx Session"=w214:T2, "AcquisitionSettings.Buffer"=w213:i32)
        n82 = for {
          N: w213 -> [_]
          tunnel: [w221] -> w204 mode=indexing
          shift-right: [w220] -> w212
          shift-left: w211 -> [w222]
          i -> [w219]
          n83 = Format Into String(format string="Stream Images %d" ("Image Name"), w219) -> (resulting string=w218:string)  [unwired: 2 in, 1 out]
          n84 = call "IMAQ Create"("Border Size"=0, "Image Name"=w218, "error in (no error)"=w222) -> ("New Image"=w221:T11, "error out"=w220:errorcluster)  [unwired: 1 in, 1 out]
        }
        n85 = call <vilib>:"IMAQdx Configure Ring Acquisition.vi"("Mode"=IMAQdx_Acquisition_Mode."Continuous" ("Continuous?"), "error in"=w212, "Images"=w204, "Session In"=w214) -> ("error out"=w206:errorcluster, "Images Out"=w208:T11[], "Session Out"=w209:T2)  [unwired: 5 in]
        n86 = Index Array(array=w208) -> (element=w207:T11)  [unwired: 1 in]
        n87 = Bundle By Name(cluster=w210, "IMAQdx Session"=w209, "Example Image"=w207, "Image Buffer"=w204) -> (w205:T14)
        n88 = Unbundle By Name(w201) -> ("VideoSave"=w200:bool)
        n89 = Select(t="FileInitialize", s=w200, f="CameraInitialize") -> (s? t:f=w199:string)
        n90 = Bundle By Name(cluster=w201, "AfterErrorCheck"=w199, "SyncWait"=FALSE, "Acquisition Configured"=TRUE) -> (w202:T10)
      }
      frame "FileInitialize " {
        n91 = Unbundle By Name(w228) -> ("FileSettings.Format"=w236:string)
        n92 = Unbundle By Name(w228) -> ("FileSettings"=w232:T22)
        n93 = Unbundle By Name(w232) -> ("FileSaveLocation"=w226:path, "FileName"=w231:string, "VideoSuffix"=w230:string)
        n94 = Concatenate Strings(w231, w230, "_0") -> (w227:string)
        n95 = case shown="\"None\"" w236 {
          tunnel: ["ErrorCheck" "InitializeIMAQ" "TDMSInitialize" "AVIInitialize"] -> w235
          tunnel: w234 -> [w239 w242 w245 w252]
          tunnel: [w238 w242 w245 w252] -> w233
          tunnel: w227 -> [_ _ w250 w254]
          tunnel: w226 -> [w237 w243 w248 w255]
          tunnel: [w237 w243 w246 w253] -> w224
          frame "BadOption", Default {
            n96 = Merge Errors(errorcluster {"status"=TRUE, "code"=199, "source"="The file format is not implemented"} ("error constant"), w239) -> (w238:errorcluster)
          }
          frame "None" {
          }
          frame "TDMS" {
            n97 = Concatenate Strings(w250, ".tdms" ("string")) -> (w247:string)
            n98 = Build Path(base path=w248, name or relative path=w247) -> (appended path=w246:path)
          }
          frame "AVI" {
            n99 = Concatenate Strings(w254, ".avi" ("string")) -> (w257:string)
            n100 = Build Path(base path=w255, name or relative path=w257) -> (appended path=w253:path)
          }
        }
        n101 = Bundle By Name(cluster=w225, "VideoPath"=w224) -> (w223:T10)
      }
      frame "AVIInitialize" {
        # "If codec selected doesn't match\nOr if user wants to select at runtime"
        # "Check Available Codecs"
        n102 = Unbundle By Name(w270) -> ("Camera Aq Attributes"=w283:T20, "Example Image"=w278:T11, "FileSettings.Codec"=w275:string, "Trigger Settings.FPS"=w259:i32, "FileSettings.Quality"=w267:i32)
        n103 = Unbundle By Name(w283) -> ("Width"=w282:u32, "Height"=w281:u32, "Format"=w280:u32, "Bit Depth"=w279:u32)
        n104 = call "GetAVICodecs.vi"("error in (no error)"=w263, "Refnum in"=w278, "Bit Depth"=w279, "Format"=w280, "Height"=w281, "Width"=w282) -> ("error out"=w274:errorcluster, "Codec Names"=w276:string[])  [unwired: 4 in]
        n105 = Search 1D Array(1D array=w276, element=w275) -> (index of element=w277:i32)  [unwired: 1 in]
        n106 = case shown="-1" w277 {
          tunnel: w276 -> [_ w289]
          tunnel: w275 -> [w285 _]
          tunnel: [w285 w288] -> w272
          tunnel: w274 -> [w284 w287]
          tunnel: [w284 w286] -> w273
          frame Default {
          }
          frame -1 {
            n107 = call "Codec Selector (SubVi).vi"("error in (no error)"=w287, "Array"=w289) -> ("error out"=w286:errorcluster, "String"=w288:string)  [unwired: 8 in]
          }
        }
        n108 = Unbundle By Name(w262) -> ("VideoPath"=w261:path)
        n109 = call "IMAQ AVI2 Create"("Quality"=w267, "error in (no error)"=w273, "Codec"=w272, "Frames Per Second"=w259, "AVI Path"=w261) -> ("error out"=w268:errorcluster, "AVI Refnum"=w269:T12)  [unwired: 5 in]
        n110 = Bundle By Name(cluster=w262, "AfterErrorCheck"="InitializeIMAQ", "FileOpen"=TRUE ("FileCreated")) -> (w266:T10)
        n111 = Bundle By Name(cluster=w270, "FileSettings.Codec"=w272, "AVIRef"=w269, "FileSettings.AVI FPS"=w259) -> (w271:T14)
      }
      frame "TDMSInitialize" {
        n112 = Unbundle By Name(w308) -> ("VideoPath"=w311:path)
        n113 = Unbundle By Name(w296) -> ("Example Image"=w312:T11, "AcquisitionSettings.FramesPerFile"=w310:i32)
        n114 = call "InitializeTDMS.vi"("FilePath"=w311, "error in (no error)"=w313, "Images per File"=w310, "Image Ref in"=w312) -> ("error out"=w298:errorcluster, "Write Settings Out"=w294:T23, "Optimizations"=w309:T24, "Refnum out"=w295:refnum<k34>)  [unwired: 4 in]
        n115 = Unbundle By Name(w308) -> ("ConfirmTDMSOptimizations"=w307:bool, "ConfirmTDMSDisableBuffer"=w303:bool)
        n116 = Bundle By Name(cluster=w296, "TDMSRef"=w295, "TDMSWSet"=w294) -> (w293:T14)
        n117 = Unbundle By Name(w309) -> ("Asynchronous Writes"=w300:bool, "Reserve Disk Space"=w299:bool, "Disable Buffering"=w291:bool)
        n118 = Not(x=w307) -> (.not. x?=w305:bool)
        n119 = Not(x=w303) -> (.not. x?=w302:bool)
        n120 = And(x=w300, y=w299) -> (x .and. y?=w306:bool)
        n121 = Or(x=w306, y=w305) -> (x .or. y?=w304:bool)
        n122 = case shown="False" w304 {
          tunnel: w300 -> [w323 _]
          tunnel: w299 -> [w324 _]
          tunnel: w298 -> [w322 w325]
          tunnel: [w321 w325] -> w297
          frame False {
            n123 = call "ShowAsynchAndReserve (SubVI).vi"("error constant 2"=w322, "Reserve Disk Space in"=w324, "Asynchronous Writes in"=w323) -> ("error constant"=w321:errorcluster)  [unwired: 6 in, 2 out]
          }
          frame True {
          }
        }
        n124 = Or(x=w291, y=w302) -> (x .or. y?=w301:bool)
        n125 = case shown="False" w301 {
          tunnel: w297 -> [w319 w320]
          tunnel: [w317 w320] -> w292
          tunnel: w291 -> [w318 _]
          frame False {
            n126 = call "Confirm Disable Buffering (SubVI).vi"("error constant 2"=w319, "Disable Buffering in"=w318) -> ("error constant"=w317:errorcluster)  [unwired: 8 in, 1 out]
          }
          frame True {
          }
        }
        n127 = Bundle By Name(cluster=w308, "AfterErrorCheck"="InitializeIMAQ", "FileOpen"=TRUE ("FileCreated")) -> (w314:T10)
      }
      frame "ErrorCheck" {
        n128 = call <extravilib>:"Write.vi"("element"=w331) -> ("channel"=w333:T25)  [unwired: 8 in, 2 out]
        n129 = call <extravilib>:"Read.vi"("channel"=w330) -> ("element"=w329:errorcluster)  [unwired: 1 in, 1 out]
        n130 = Merge Errors(w329, w331) -> (w332:errorcluster)
        n131 = Unbundle By Name(w327) -> ("AfterErrorCheck"=w336:string)
        n132 = flat-sequence {
          tunnel: w336 -> [w341]
          tunnel: "Shutdown" ("t") -> [w340]
          tunnel: w332 -> [w338]
          tunnel: [w339] -> w328
          tunnel: [w345] -> w334
          tunnel: w328 -> [w345]
          tunnel: w327 -> [w344]
          tunnel: [w342] -> w326
          frame #0 {
            n133 = Select(t=w340, s=w338, f=w341) -> (s? t:f=w339:string)
          }
          frame #1 {
            n134 = Bundle By Name(cluster=w344, "AfterErrorCheck"="Shutdown") -> (w342:T10)
          }
        }
      }
      frame "InitializeIMAQ" {
        n135 = Unbundle By Name(w346) -> ("IMAQdx Session"=w349:T2)
        n136 = call <vilib>:"IMAQdx Start Acquisition.vi"("error in"=w351, "Session In"=w349) -> ("error out"=w350:errorcluster, "Session Out"=w348:T2)  [unwired: 8 out]
        n137 = Bundle By Name(cluster=w352, "AfterErrorCheck"="InitializeCameraTrigger", "AcquisitionStarted"=TRUE ("FileCreated")) -> (w353:T10)
        n138 = Bundle By Name(cluster=w346, "IMAQdx Session"=w348) -> (w347:T14)
      }
      frame "InitializeCameraTrigger" {
        n139 = Unbundle By Name(w360) -> ("Trigger Settings"=w371:T21, "Camera Attributes.Exposure Start Delay"=w367:dbl)
        n140 = Unbundle By Name(w371) -> ("FPS"=w370:i32, "Exposure Time"=w369:dbl, "Start Trigger Source"=w368:tag, "Camera\nClock\nCounter"=w365:tag, "PhysicalCameraSignalLine"=w364:tag, "Sync Type"=w363:T26)
        n141 = call "CameraTriggerSetup.vi"("Camera\nTrigger\nOutput"=w364, "Frame Rate"=w370, "Sync Type"=w363, "Exposure Time"=w369, "error in"=w366, "Camera\nClock\nCounter"=w365, "Start Trigger Source"=w368, "Exposure Start Delay"=w367) -> ("error out"=w362:errorcluster, "CameraSignalDefinition"=w358:T27, "CameraSignalRefnum"=w359:refnum<k21>)  [unwired: 1 in]
        n142 = Bundle By Name(cluster=w360, "CameraSignalRefnum"=w359, "CameraSignalDefinition"=w358) -> (w361:T14)
      }
      frame "WaitForAcStart" {
        # "Counter output can never be the origin of a start trigger,\ninitializing it first always works."
        n143 = Unbundle By Name(w379) -> ("CameraSignalRefnum"=w386:refnum<k21>)
        n144 = Unbundle By Name(w382) -> ("SyncStart"=w388:bool)
        n145 = call <vilib>:"DAQmx Start Task.vi"("task/channels in"=w386, "error in"=w385) -> ("task out"=w384:refnum<k21>, "error out"=w387:errorcluster)  [unwired: 12 in]
        n146 = case shown="True" w388 {
          tunnel: w387 -> [w389 w401]
          tunnel: [w389 w396] -> w377
          tunnel: w379 -> [_ w405]
          tunnel: [_ w391] -> w374
          tunnel: w373 -> [_ w393]
          frame False {
          }
          frame True {
            w403 = tag "/Dev1/ao/StartTrigger"  # Output Start Trigger
            w404 = tag "/Dev1/ai/StartTrigger"  # Input Start Trigger
            n147 = Unbundle By Name(w405) -> ("Trigger Settings.Start Trigger Source"=w402:tag)
            n148 = Equal?(x=w404, y=w402) -> (x = y?=w397:bool)
            n149 = Equal?(x=w403, y=w402) -> (x = y?=w398:bool)
            n150 = Not Or(1:w397, 2:w398) -> (0:w399:bool)
            n151 = case shown="True" w399 {
              tunnel: [errorcluster {"status"=FALSE, "code"=0, "source"=""} ("error constant") errorcluster {"status"=TRUE, "code"=501, "source"="Trigger source doesn't match expected options"} ("error constant")] -> w400
              frame False {
              }
              frame True {
              }
            }
            n152 = Merge Errors(w401, w400) -> (w390:errorcluster)
            n153 = case shown="Error .." w390 {
              tunnel: ["Start" "Abort"] -> w392
              frame No Error {
              }
              frame Error {
              }
            }
            n154 = call <extravilib>:"Write.vi"("element"=w392) -> ("channel"=w391:T28)  [unwired: 8 in, 2 out]
            n155 = call <extravilib>:"Read.vi"("channel"=w393) -> ("element"=w395:string)  [unwired: 1 in, 1 out]
            n156 = case shown="\"Start\"" w395 {
              tunnel: [errorcluster {"status"=TRUE, "code"=105, "source"="Other\nChannel Stopped"} ("error constant") errorcluster {"status"=FALSE, "code"=0, "source"=""} ("error constant")] -> w394
              frame "Abort", Default {
              }
              frame "Start" {
              }
            }
            n157 = Merge Errors(w390, w394) -> (w396:errorcluster)
          }
        }
        n158 = Bundle By Name(cluster=w379, "CameraSignalRefnum"=w384) -> (w383:T14)
        n159 = Bundle By Name(cluster=w382, "TriggerStarted"=TRUE) -> (w381:T10)
        n160 = Select(t="ErrorCheck", s=w377, f="Acquire" ("AfterErrorCheck")) -> (s? t:f=w378:string)
      }
      frame "Acquire" {
        w417 = T29 0 items=["no dialog", "OK message", "continue or stop message", "OK message + warnings", "continue/stop + warnings"] ("type of dialog (OK msg:1)")
        w418 = 1 items=["no exception", "cancel error on match", "set error on match"] ("[exception action] (none:0)")
        w448 = errorcluster {"status"=FALSE, "code"=0, "source"=""}  # Initial Value
        w447 = T11 refnum ("Image Out")
        w457 = FALSE  # Release Previous
        # "Only shutdown image acquisition\non timeout or error"
        # "Exclude timout error"
        # "Check if generation error"
        n161 = Unbundle By Name(w413) -> ("IMAQdx Session"=w412:T2)
        n162 = feedback #1(u32 0) -> (w451:u32)
        n163 = call <vilib>:"IMAQdx Extract Image.vi"("Release Previous (true)"=w457, "Buffer Number Mode (Next)"=IMAQdx_Buffer_Number_Mode."Buffer Number" ("Buffer Number Mode"), "error in"=w450, "Buffer Number In"=w451, "Session In"=w412) -> ("error out"=w449:errorcluster, "Buffer Number Out"=w452:u32, "Image Out"=w453:T11, "Session Out"=w434:T2)  [unwired: 3 in]
        n164 = Compound Arithmetic op=ADD(u32 1 ("value"), w452) -> (w456:u32)
        n165 = feedback-in #1(w456) -> ()
        n166 = feedback #2(w448) -> (w430:errorcluster)
        n167 = feedback-in #2(w449) -> ()
        n168 = call <vilib>:"IMAQdx Calculate Frames per Second.vi"("Session In"=w434, "Buffer Number"=w452) -> ()  [unwired: 7 in, 7 out]
        n169 = feedback #3(w447) -> (w445:T11)
        n170 = feedback-in #3(w453) -> ()
        n171 = Bundle By Name(cluster=cluster{"Image":T11, "Session":T2} {"Image"=refnum, "Session"=""}, "Image"=w445, "Session"=w434) -> (w438:cluster{"Image":T11, "Session":T2})
        n172 = Not Equal?(x=w445, y=w447) -> (x != y?=w414:bool)
        n173 = case shown="True" w414 {
          tunnel: w430 -> [w476 w489]
          tunnel: [w476 w487] -> w416
          tunnel: w413 -> [w475 w490]
          tunnel: w438 -> [_ w482]
          tunnel: [w475 w480] -> w444
          frame False {
          }
          frame True {
            n174 = Unbundle By Name(w490) -> ("AcquisitionSettings.FramesPerFile"=w495:i32, "FileSettings.Format"=w485:string)
            n175 = feedback #4(0) -> (w491:i32)
            n176 = Equal?(x=w491, y=w495) -> (x = y?=w494:bool)
            n177 = case shown="True" w494 {
              tunnel: [w515 1] -> w492
              tunnel: w491 -> [w516 _]
              tunnel: w485 -> [_ w521]
              tunnel: w490 -> [w514 w520]
              tunnel: w489 -> [w513 w519]
              tunnel: [w513 w518] -> w486
              tunnel: [w514 w517] -> w481
              frame False {
                n178 = Increment(x=w516) -> (x+1=w515:i32)
              }
              frame True {
                n179 = case shown="\"AVI\"" w521 {
                  tunnel: w520 -> [w526 w530 w539]
                  tunnel: w519 -> [w528 w529 w541]
                  tunnel: [w524 w529 w532] -> w518
                  tunnel: [w523 w530 w543] -> w517
                  frame "TDMS", Default {
                    n180 = Unbundle By Name(w526) -> ("TDMSRef"=w527:refnum<k34>)
                    n181 = call "TDMS Start New File.vi"("error in"=w528, "Previous TDMS Refnum In"=w527) -> ("error out"=w524:errorcluster, "New TDMS Refnum Out"=w525:refnum<k34>)  [unwired: 8 in]
                    n182 = Bundle By Name(cluster=w526, "TDMSRef"=w525) -> (w523:T14)
                  }
                  frame "None" {
                  }
                  frame "AVI" {
                    n183 = Unbundle By Name(w539) -> ("AVIRef"=w542:T12)
                    n184 = call "IMAQ AVI2 Close"("error in (no error)"=w541, "AVI Refnum"=w542) -> ("error out"=w540:errorcluster)  [unwired: 9 in]
                    n185 = Unbundle By Name(w539) -> ("FileSettings"=w538:T22)
                    n186 = Unbundle By Name(w538) -> ("FileSaveLocation"=w536:path, "AVI FPS"=w535:i32, "Codec"=w534:string, "Quality"=w533:i32)
                    n187 = call "Increment Filename.vi"("Path In"=w536) -> ("Incremented Path Out"=w537:path)  [unwired: 10 in]
                    n188 = call "IMAQ AVI2 Create"("Quality"=w533, "error in (no error)"=w540, "Codec"=w534, "Frames Per Second"=w535, "AVI Path"=w537) -> ("error out"=w532:errorcluster, "AVI Refnum"=w531:T12)  [unwired: 5 in]
                    n189 = Bundle By Name(cluster=w539, "AVIRef"=w531) -> (w543:T14)
                  }
                }
              }
            }
            n190 = feedback-in #4(w492) -> ()
            n191 = Unbundle By Name(w482) -> ("Session"=w478:T2, "Image"=w477:T11)
            n192 = call "High Resolution Timer Helper.vi"("error in (no error)"=w486) -> ("error out"=w484:errorcluster, "Current Time"=w479:dbl)  [unwired: 8 in, 1 out]
            n193 = case shown="\"TDMS\"" w485 {
              tunnel: w484 -> [w497 w504 w512]
              tunnel: [w497 w503 w511] -> w483
              tunnel: w477 -> [_ w502 w510]
              tunnel: w481 -> [w496 w499 w506]
              tunnel: [w496 w498 w507] -> w480
              frame "None", Default {
              }
              frame "AVI" {
                n194 = Unbundle By Name(w499) -> ("AVIRef"=w501:T12)
                n195 = call "IMAQ AVI2 Write Frame"("error in (no error)"=w504, "Image"=w502, "AVI Refnum"=w501) -> ("error out"=w503:errorcluster, "AVI Refnum (duplicate)"=w500:T12)  [unwired: 6 in, 1 out]
                n196 = Bundle By Name(cluster=w499, "AVIRef"=w500) -> (w498:T14)
              }
              frame "TDMS" {
                n197 = Unbundle By Name(w506) -> ("TDMSRef"=w509:refnum<k34>, "TDMSWSet"=w508:T23)
                n198 = call "TDMS Write File.vi"("error in"=w512, "Write Settings"=w508, "Image"=w510, "TDMS Ref In"=w509) -> ("error out"=w511:errorcluster, "TDMS Ref Out"=w505:refnum<k34>)  [unwired: 6 in]
                n199 = Bundle By Name(cluster=w506, "TDMSRef"=w505) -> (w507:T14)
              }
            }
            n200 = call "High Resolution Timer Helper.vi"("error in (no error)"=w483, "Previous Time"=w479) -> ("error out"=w488:errorcluster)  [unwired: 7 in, 2 out]
            n201 = call <vilib>:"IMAQdx Release Image.vi"("error in"=w488, "Image"=w477, "Session In"=w478) -> ("error out"=w487:errorcluster)  [unwired: 7 in, 1 out]
          }
        }
        n202 = Unbundle By Name(w413) -> ("DisplayEveryNFrames"=w441:i32)
        n203 = feedback #5(0) -> (w440:i32)
        n204 = Equal?(x=w441, y=w440) -> (x = y?=w442:bool)
        n205 = case shown="True" w442 {
          tunnel: w440 -> [w470 _]
          tunnel: [w469 1] -> w439
          tunnel: w438 -> [_ w473]
          tunnel: [_ w471] -> w437
          frame False {
            n206 = Increment(x=w470) -> (x+1=w469:i32)
          }
          frame True {
            n207 = Unbundle By Name(w473) -> ("Image"=w472:T11)
            n208 = call <extravilib>:"Write.vi"("element"=w472) -> ("channel"=w471:T30)  [unwired: 1 out]
          }
        }
        n209 = feedback-in #5(w439) -> ()
        n210 = Unbundle By Name(w430) -> ("code"=w429:i32)
        n211 = Unbundle By Name(w413) -> ("CameraSignalRefnum"=w431:refnum<k21>)
        n212 = Equal?(x=-1074396030, y=w429) -> (x = y?=w420:bool)
        n213 = case shown="True" w420 {
          tunnel: ["Acquire" ("AfterErrorCheck") "Shutdown"] -> w432
          frame False {
          }
          frame True {
          }
        }
        n214 = call <extravilib>:"Read.vi"("channel"=w433) -> ("element"=w427:bool)  [unwired: 1 in, 1 out]
        n215 = call <vilib>:"DAQmx Is Task Done.vi"("task/channels in"=w431) -> ("task out"=w424:refnum<k21>, "task done?"=w426:bool, "error out"=w423:errorcluster)  [unwired: 12 in]
        n216 = Or(x=w427, y=w426) -> (x .or. y?=w425:bool)
        n217 = case shown="False" w425 {
          tunnel: w424 -> [_ w464]
          tunnel: w423 -> [_ w463]
          tunnel: w422 -> [w459 w462]
          tunnel: [w459 w460] -> w421
          frame False {
          }
          frame True {
            # "If stopped or signal error\nNeed to shut down signal\nimmediately to let buffer catch up"
            n218 = call <vilib>:"DAQmx Stop Task.vi"("task/channels in"=w464, "error in"=w463) -> ("task out"=w466:refnum<k21>, "error out"=w465:errorcluster)  [unwired: 12 in]
            n219 = call <vilib>:"DAQmx Clear Task.vi"("task in"=w466, "error in"=w465) -> ()  [unwired: 13 in, 1 out]
            n220 = Bundle By Name(cluster=w462, "TriggerStarted"=FALSE) -> (w460:T10)
          }
        }
        n221 = call <vilib>:"General Error Handler.vi"("type of dialog (OK msg:1)"=w417, "error in (no error)"=w416, "[exception action] (none:0)"=w418, "[exception code]"=-1074396030 ("x")) -> ("error out"=w415:errorcluster)  [unwired: 7 in, 4 out]
        n222 = Select(t="ErrorCheck", s=w415, f=w432) -> (s? t:f=w435:string)
      }
      frame "Shutdown" {
        n223 = Unbundle By Name(w546) -> ("ShutdownActions"=w544:string[])
        n224 = Empty Array?(array=w544) -> (empty?=w545:bool)
        n225 = case shown="True" w545 {
          tunnel: w546 -> [_ w562]
          tunnel: [w553 w560] -> w549
          tunnel: w544 -> [w553 w561]
          frame False {
          }
          frame True {
            n226 = Unbundle By Name(w562) -> ("TriggerStarted"=w569:bool, "AcquisitionStarted"=w568:bool, "Acquisition Configured"=w567:bool, "FileOpen"=w566:bool, "CameraOpen"=w565:bool, "BufferOpen"=w558:bool)
            n227 = Build Array(w569, w568, w567, w566, w565, w558) -> (w563:bool[])
            n228 = Build Array("ShutdownTrigger", "ShutdownAcquisition", "Unconfigure Acquisition", "CloseFile", "ShutdownCamera", "ReleaseBuffer") -> (w564:string[])
            n229 = for {
              tunnel: w564 -> [w574] mode=indexing
              tunnel: w563 -> [w575] mode=indexing
              shift-right: [w572] -> w560
              shift-left: w561 -> [w573]
              n230 = case shown="True" w575 {
                tunnel: w574 -> [_ w579]
                tunnel: w573 -> [w576 w578]
                tunnel: [w576 w577] -> w572
                frame False {
                }
                frame True {
                  n231 = Insert Into Array(array=w578, new element=w579) -> (w577:string[])  [unwired: 1 in]
                }
              }
            }
            n232 = Insert Into Array(array=w560, new element="FinalErrorHandler" ("new element/subarray")) -> ()  [unwired: 1 in, 1 out]
          }
        }
        n233 = Delete From Array(array=w549) -> (deleted portion=w548:string, array with subset deleted=w547:string[])  [unwired: 2 in]
        n234 = Bundle By Name(cluster=w546, "ShutdownActions"=w547) -> (w552:T10)
      }
      frame "ShutdownTrigger " {
        n235 = Unbundle By Name(w583) -> ("CameraSignalRefnum"=w586:refnum<k21>)
        n236 = call <vilib>:"DAQmx Stop Task.vi"("task/channels in"=w586, "error in"=w585) -> ("task out"=w589:refnum<k21>, "error out"=w588:errorcluster)  [unwired: 12 in]
        n237 = call <vilib>:"DAQmx Clear Task.vi"("task in"=w589, "error in"=w588) -> ("error out"=w584:errorcluster)  [unwired: 13 in]
        n238 = Bundle By Name(cluster=w582, "TriggerStarted"=FALSE) -> (w581:T10)
      }
      frame "ShutdownAcquisition" {
        n239 = Unbundle By Name(w597) -> ("IMAQdx Session"=w599:T2)
        n240 = call <vilib>:"IMAQdx Stop Acquisition.vi"("error in"=w595, "Session In"=w599) -> ("error out"=w594:errorcluster, "Session Out"=w598:T2)  [unwired: 8 out]
        n241 = Bundle By Name(cluster=w597, "IMAQdx Session"=w598) -> (w596:T14)
        n242 = Bundle By Name(cluster=w592, "AcquisitionStarted"=FALSE) -> (w590:T10)
      }
      frame "UnconfigureAcquisition" {
        n243 = Unbundle By Name(w606) -> ("IMAQdx Session"=w608:T2)
        n244 = call <vilib>:"IMAQdx Unconfigure Acquisition.vi"("error in"=w602, "Session In"=w608) -> ("error out"=w603:errorcluster, "Session Out"=w607:T2)  [unwired: 8 out]
        n245 = Bundle By Name(cluster=w606, "IMAQdx Session"=w607) -> (w605:T14)
        n246 = Bundle By Name(cluster=w601, "Acquisition Configured"=FALSE) -> ()  [unwired: 1 out]
      }
      frame "CloseFile" {
        n247 = Unbundle By Name(w612) -> ("FileSettings.Format"=w614:string)
        n248 = case shown="\"None\"" w614 {
          tunnel: w616 -> [w620 w624 w626]
          tunnel: [w617 w623 w626] -> w615
          tunnel: w612 -> [w619 w622 _]
          frame "AVI", Default {
            n249 = Unbundle By Name(w619) -> ("AVIRef"=w618:T12)
            n250 = call "IMAQ AVI2 Close"("error in (no error)"=w620, "AVI Refnum"=w618) -> ("error out"=w617:errorcluster)  [unwired: 9 in]
          }
          frame "TDMS" {
            n251 = Unbundle By Name(w622) -> ("TDMSRef"=w621:refnum<k34>)
            n252 = TDMS Advanced Close(6:10.0 ("timeout (10 s)"), 8:w624, 11:w621) -> (0:w623:errorcluster)  [unwired: 1 in, 1 out]
          }
          frame "None" {
          }
        }
        n253 = Bundle By Name(cluster=w611, "FileOpen"=FALSE ("FileCreated")) -> (w610:T10)
      }
      frame "ShutdownCamera" {
        n254 = Unbundle By Name(w633) -> ("IMAQdx Session"=w634:T2)
        n255 = call <vilib>:"IMAQdx Close Camera.vi"("error in"=w632, "Session In"=w634) -> ("error out"=w631:errorcluster)  [unwired: 9 out]
        n256 = Bundle By Name(cluster=w629, "CameraOpen"=FALSE) -> (w627:T10)
      }
      frame "ReleaseBuffer" {
        n257 = Unbundle By Name(w639) -> ("Image Buffer"=w641:T11[])
        n258 = for {
          shift-right: [w643] -> _
          shift-left: _ -> [w644]
          tunnel: w641 -> [w642] mode=indexing
          n259 = call "IMAQ Dispose"("Image"=w642, "error in (no error)"=w644) -> ("error out"=w643:errorcluster)  [unwired: 4 in]
        }
        n260 = Bundle By Name(cluster=w637, "BufferOpen"=FALSE) -> (w635:T10)
      }
      frame "FinalErrorHandler" {
        n261 = call <vilib>:"Simple Error Handler.vi"("error in (no error)"=w651) -> ("error out"=w647:errorcluster)  [unwired: 4 in, 4 out]
        n262 = property on="Cluster - Borderless" class="Clust (strict)"(error in=w647, "DisabledEnum"=T16."Enabled" ("Disabled")) -> (error out=w646:errorcluster)  [unwired: 1 in, 1 out]
      }
    }
  }
  n263 = while {
    shift-right: [w662] -> _
    shift-left: _ -> [w661]
    shift-right: [w659] -> _
    shift-left: _ -> [w658]
    shift-right: [w657] -> _
    shift-left: T9 {"Physical Settings"={"physical channels"="Dev1/ao0:2", "source"="OnboardClock", "Start Trigger"="/Dev1/ai/StartTrigger", "StartTriggered"=TRUE}, "OutputTask"="", "GenerationSettings"={"NumberOfSamples"=100000, "Sample Rate"=0}, "Channel Names"=""} -> [w660]
    shift-right: [w655] -> _
    shift-left: w32 -> [w656]
    tunnel: w31 -> [w654]
    tunnel: [w653] -> w30
    stop <- "Stop 7" stop-if-true
    # "Analog Output"
    n264 = case shown="\"Idle\", Default" w661 {
      tunnel: ["InitializeSignal" "WaitForAcStart" w707 "Temp" w816] -> w662
      tunnel: w660 -> [w667 w689 w715 w798 w814]
      tunnel: [w671 w691 w713 w796 w813] -> w659
      tunnel: w658 -> [w670 w699 w717 w805 w813]
      tunnel: [w668 w690 w714 w799 w814] -> w657
      tunnel: w656 -> [w665 w695 w706 w803 w815]
      tunnel: [w665 w693 w706 w801 w815] -> w655
      tunnel: [_ _ w709 _ _] -> w654
      tunnel: [_ _ w710 _ _] -> w653
      frame "InitializeChannels" {
        n265 = Unbundle By Name(w667) -> ("Physical Settings"=w676:T31, "Channel Names"=w664:string, "GenerationSettings.Sample Rate"=w663:i32)
        n266 = Unbundle By Name(w676) -> ("Start Trigger"=w674:tag, "source"=w673:tag, "physical channels"=w675:tag, "StartTriggered"=w672:bool)
        n267 = call-poly <vilib>:"DAQmx Create Virtual Channel.vi"("physical channels"=w675, "name to assign"=w664, "error in"=w670) -> ("task out"=w679:refnum<k21>, "error out"=w680:errorcluster)  [unwired: 11 in]
        n268 = call-poly <vilib>:"DAQmx Timing.vi"("task/channels in"=w679, "rate"=w663, "source"=w673, "error in"=w680) -> ("task out"=w678:refnum<k21>, "error out"=w677:errorcluster)  [unwired: 10 in]
        n269 = case shown="False" w672 {
          tunnel: w678 -> [w681 w687]
          tunnel: w677 -> [w682 w686]
          tunnel: w674 -> [_ w685]
          tunnel: [w682 w683] -> w671
          tunnel: [w681 w684] -> w666
          frame False {
          }
          frame True {
            n270 = call-poly <vilib>:"DAQmx Trigger.vi"("task/channels in"=w687, "source"=w685, "error in"=w686) -> ("task out"=w684:refnum<k21>, "error out"=w683:errorcluster)  [unwired: 11 in]
          }
        }
        n271 = Bundle By Name(cluster=w667, "OutputTask"=w666) -> (w668:T9)
      }
      frame "InitializeSignal" {
        n272 = Unbundle By Name(w689) -> ("GenerationSettings.NumberOfSamples"=w698:i32, "OutputTask"=w697:refnum<k21>)
        n273 = property class="DAQmx Timing"(reference=w697, error in=w699) -> (reference out=w700:refnum<k21>, error out=w703:errorcluster, "SampClk.Rate"=w704:dbl)
        n274 = Unbundle By Name(w695) -> ("PreviousInfo"=w696:T32)
        n275 = property on="Outputs" class="Clust (strict)"() -> ("Value"=w705:T33)  [unwired: 2 in, 2 out]
        n276 = call "GenerateOutputSignal (SubVI).vi"("PreviousInfoIn"=w696, "error constant"=w703, "#s"=w698, "Fs"=w704, "Outputs"=w705) -> ("error constant 2"=w702:errorcluster, "PreviousInfoOut"=w694:T32, "Waveforms"=w701:waveform(dbl)[])  [unwired: 4 in]
        n277 = Bundle By Name(cluster=w695, "PreviousInfo"=w694) -> (w693:T8)
        n278 = call-poly <vilib>:"DAQmx Write.vi"("task/channels in"=w700, "data"=w701, "error in"=w702) -> ("task out"=w688:refnum<k21>, "error out"=w691:errorcluster)  [unwired: 10 in, 1 out]
        n279 = Bundle By Name(cluster=w689, "OutputTask"=w688) -> (w690:T9)
      }
      frame "WaitForAcStart" {
        n280 = Unbundle By Name(w706) -> ("SyncStart"=w719:bool, "Leader"=w712:bool, "NoDependants"=w711:i32)
        n281 = Unbundle By Name(w715) -> ("OutputTask"=w718:refnum<k21>)
        n282 = case shown="True" w719 {
          tunnel: w718 -> [w726 w734]
          tunnel: w717 -> [w725 w735]
          tunnel: [w724 w732] -> w716
          tunnel: [w723 w733] -> w713
          tunnel: w712 -> [_ w736]
          tunnel: w709 -> [_ w731]
          tunnel: w711 -> [_ w730]
          tunnel: [_ w729] -> w710
          tunnel: [_ w728] -> w709
          tunnel: ["Start" ("element") w727] -> w708
          frame False {
            n283 = call <vilib>:"DAQmx Start Task.vi"("task/channels in"=w726, "error in"=w725) -> ("task out"=w724:refnum<k21>, "error out"=w723:errorcluster)  [unwired: 12 in]
          }
          frame True {
            n284 = case shown="False" w736 {
              tunnel: w735 -> [w743 w756]
              tunnel: w734 -> [w742 w757]
              tunnel: [w741 w754] -> w733
              tunnel: [w740 w755] -> w732
              tunnel: w731 -> [_ w760]
              tunnel: w730 -> [_ w759]
              tunnel: [w738 w753] -> w729
              tunnel: [w739 _] -> w728
              tunnel: [w737 w752] -> w727
              frame False {
                n285 = flat-sequence {
                  tunnel: w743 -> [w747]
                  tunnel: w742 -> [w746]
                  tunnel: [w745] -> w741
                  tunnel: [w744] -> w740
                  tunnel: [w748] -> w739
                  tunnel: [w751] -> w738
                  tunnel: [w750] -> w737
                  frame #0 {
                    n286 = call <vilib>:"DAQmx Start Task.vi"("task/channels in"=w746, "error in"=w747) -> ("task out"=w744:refnum<k21>, "error out"=w745:errorcluster)  [unwired: 12 in]
                  }
                  frame #1 {
                    n287 = call <extravilib>:"Write.vi"("element"="Start") -> ("channel"=w748:T28)  [unwired: 8 in, 2 out]
                  }
                  frame #2 {
                    n288 = call <extravilib>:"Read.vi"() -> ("channel"=w751:T34, "element"=w750:string)  [unwired: 1 in, 1 out]
                  }
                }
              }
              frame True {
                n289 = flat-sequence {
                  tunnel: w760 -> [w764]
                  tunnel: w759 -> [w762]
                  tunnel: [w761] -> w758
                  tunnel: w758 -> [w786]
                  tunnel: w757 -> [w785]
                  tunnel: w756 -> [w784]
                  tunnel: [w783] -> w755
                  tunnel: [w782] -> w754
                  tunnel: [w781] -> w753
                  tunnel: [w780] -> w752
                  frame #0 {
                    n290 = while {
                      tunnel: w764 -> [w777]
                      shift-right: [w770] -> _
                      shift-left: 0 -> [w771]
                      tunnel: w762 -> [w769]
                      tunnel: [w765] -> w761
                      stop <- w767 stop-if-true
                      n291 = call <extravilib>:"Read.vi"("channel"=w777) -> ("element"=w775:string)  [unwired: 8 in, 2 out]
                      n292 = Equal?(x="Start", y=w775) -> (x = y?=w773:bool)
                      n293 = Increment(x=w771) -> (x+1=w772:i32)
                      n294 = Equal?(x="Abort", y=w775) -> (x = y?=w766:bool)
                      n295 = Select(t=w772, s=w773, f=w771) -> (s? t:f=w770:i32)
                      n296 = Equal?(x=w770, y=w769) -> (x = y?=w768:bool)
                      n297 = Or(x=w766, y=w768) -> (x .or. y?=w767:bool)
                      n298 = case shown="True" w766 {
                        tunnel: ["Start" "Abort"] -> w765
                        frame False {
                        }
                        frame True {
                        }
                      }
                    }
                  }
                  frame #1 {
                    n299 = case shown="\"Start\"" w786 {
                      tunnel: w785 -> [w788 w794]
                      tunnel: w784 -> [w787 w793]
                      tunnel: [w788 w792] -> w783
                      tunnel: [w787 w791] -> w782
                      tunnel: ["Abort" "Start"] -> w780
                      frame "Abort", Default {
                      }
                      frame "Start" {
                        n300 = call <vilib>:"DAQmx Start Task.vi"("task/channels in"=w794, "error in"=w793) -> ("task out"=w792:refnum<k21>, "error out"=w791:errorcluster)  [unwired: 12 in]
                      }
                    }
                    n301 = call <extravilib>:"Write.vi"("element"=w780) -> ("channel"=w781:T34)  [unwired: 1 out]
                  }
                }
              }
            }
          }
        }
        n302 = Bundle By Name(cluster=w715, "OutputTask"=w716) -> (w714:T9)
        n303 = case shown="\"Start\"" w708 {
          tunnel: ["Shutdown" "Generate"] -> w707
          frame "Abort", Default {
          }
          frame "Start" {
          }
        }
      }
      frame "Generate" {
        n304 = Unbundle By Name(w798) -> ("GenerationSettings.NumberOfSamples"=w807:i32, "OutputTask"=w806:refnum<k21>)
        n305 = property class="DAQmx Timing"(reference=w806, error in=w805) -> (reference out=w808:refnum<k21>, error out=w811:errorcluster, "SampClk.Rate"=w812:dbl)
        n306 = Unbundle By Name(w803) -> ("PreviousInfo"=w804:T32)
        n307 = property on="Outputs" class="Clust (strict)"() -> ("Value"=w800:T33)  [unwired: 2 in, 2 out]
        n308 = call "GenerateOutputSignal (SubVI).vi"("PreviousInfoIn"=w804, "error constant"=w811, "#s"=w807, "Fs"=w812, "Outputs"=w800) -> ("error constant 2"=w810:errorcluster, "PreviousInfoOut"=w802:T32, "Waveforms"=w809:waveform(dbl)[])  [unwired: 4 in]
        n309 = Bundle By Name(cluster=w803, "PreviousInfo"=w802) -> (w801:T8)
        n310 = call-poly <vilib>:"DAQmx Write.vi"("task/channels in"=w808, "data"=w809, "error in"=w810) -> ("task out"=w797:refnum<k21>, "error out"=w796:errorcluster)  [unwired: 10 in, 1 out]
        n311 = Bundle By Name(cluster=w798, "OutputTask"=w797) -> (w799:T9)
      }
      frame "Idle", Default {
        n312 = event shown="[1] \"Re/Start Acquisition\": Value Change" {
          selector: _ -> [_ _]
          dyn-events: _ -> [_ _]
          timeout: _ -> [_ _]
          tunnel: [_ w818] -> w816
          tunnel: "InitializeChannels" -> [_ w818]
          event Timeout {
            n313 = event-data() -> ()  [unwired: 1 in, 3 out]
          }
          event "Re/Start Acquisition": Value Change {
            n314 = event-data() -> ()  [unwired: 1 in, 6 out]
          }
        }
      }
    }
  }
  n315 = while {
    tunnel: w39 -> [w824]
    shift-right: [w822] -> _
    shift-left: errorcluster {"status"=FALSE, "code"=0, "source"=""} ("error IO") -> [w821]
    tunnel: [w820] -> w37
    stop <- "Stop 3" stop-if-true
    n316 = call <extravilib>:"Read.vi"("channel"=w824) -> ("element"=w823:errorcluster)  [unwired: 8 in, 2 out]
    n317 = Merge Errors(w821, w823) -> (w822:errorcluster)
    n318 = call <extravilib>:"Write.vi"("element"=w822) -> ("channel"=w820:T35)  [unwired: 1 out]
  }
  n319 = while {
    tunnel: w36 -> [w826]
    tunnel: w35 -> [w828]
    stop <- w827 stop-if-true
    n320 = call <extravilib>:"Read.vi"("channel"=w826) -> ("element"=w825:T11)  [unwired: 1 in, 1 out]
    n321 = call "CameraDisplay.vi"("Image Display 2"=w825) -> ()  [unwired: 10 in, 1 out]
    n322 = call <extravilib>:"Read.vi"("channel"=w828) -> ("element"=w827:bool)  [unwired: 1 in, 1 out]
  }
